vi "RG TAS v4c_Jamie_PIA.vi"() -> ()   [LabVIEW 2015]
uses:
  <vilib>/Analysis/2dsp.llb/Decimate (single shot, DBL).vi
  <vilib>/DAQmx/read.llb/DAQmx Read (Analog Wfm 1Chan NSamp).vi
  <vilib>/Analysis/baseanly.llb/Mean (DBL).vi
  Chaz TAS - DR/Sub VIs/Mono/global_Test.vi
  <vilib>/Instr/_visa.llb/VISA Configure Serial Port (Instr).vi
  Sub VIs/global tas.vi
  <vilib>/DAQmx/miscellaneous.llb/DAQmx Fill In Error Info.vi
  <vilib>/Utility/file.llb/Write To Spreadsheet File (DBL).vi
  <vilib>/Waveform/WDTOps.llb/WDT Index Channel DBL.vi
  <vilib>/Utility/file.llb/Write Delimited Spreadsheet (DBL).vi
  Program Files/National Instruments/LabVIEW 2014/instr.lib/Tektronix DPO MSO 2000 4000 Series/Tektronix DPO MSO 2000 4000 Series.lvlib
  <vilib>/Analysis/NI_AALPro.lvlib
  <vilib>/Analysis/NI_AALBase.lvlib
panel:
  in  "Inspect Traces":bool
  out "DAQ Loop":i32
  out "Scope Error Counter":i32
  out "Scope time axis":dbl[](array[numeric])
  in  "Stop acquisition":bool
  out "Grating":i32
  in  "2b - Spectrum":bool
  in  "2a - Kinetic":bool
  in  "Stop":bool
  out "Btrace Readout Counter":i32=2
  in  "Stop Btrace Measurement":bool
  out "Readout Counter":i32=2
  in  "Stop Measurement":bool
  in  "Calculate Output Method":T1(ring)=enum."Reflectance"
  in  "Parameters":T2(tab)
  in  "Shutter flow control":u16(ring) items=["None"=0, "XON/XOFF"=1, "RTS/CTS"=2, "DTR/DSR"=4]
  in  "Shutter stop bits":u16(ring)=10 items=["1.0"=10, "1.5"=15, "2.0"=20]
  in  "Shutter parity":u16(ring) items=["None", "Odd", "Even", "Mark", "Space"]
  in  "Shutter data bits":u16=8 min=5 max=8 step=1
  in  "Shutter VISA resource name":refnum<visa-resource-name>="COM1"
  in  "Shutter baud rate":u32=9600
  in  "Shutter open string":string="+100 10\n"
  in  "1 - Move Shutter":bool
  in  "3 - Move mono":bool
  out "Current wavelength (Oriel)":dbl format="%#_13g"
  in  "Monochromator Type":bool=TRUE
  out "Start Wavelength":dbl min=0.0 format="%.3f"
  out "End Wavelength":dbl=100.0 min=0.0 format="%.3f"
  out "Interval Wavelength":dbl=10.0 min=0.0 format="%.3f"
  out "Current Wavelength (PTI)":dbl=300.0 min=300.0 max=2000.0 step=1.0
  in  "Is IR":bool caption="Grating"
  in  "Mono VISA name":refnum<visa-resource-name>
  in  "Mono 2 VISA name":refnum<visa-resource-name>
  out "DAQ dt":dbl=5e-06
  in  "DAQ End Time (s)":dbl=1.0
  in  "DAQ rate":i32=1250000
  in  "DAQ Trigger Level (V)":dbl=0.2
  out "DAQ Number of Samples":dbl=10000.0
  in  "DAQ average number of points":dbl=50.0
  out "DAQ final number of points":dbl
  in  "DAQ Input Channel":tag="Dev1/ai0"
  in  "100% Reflectance Standard (V)":dbl=1.0
  in  "DAQ Card":enum16{"USB-6211", "USB-6251"}(ring)=enum."USB-6251"
  in  "DAQ Input Config":i32(ring)=10106 items=["default"=-1, "RSE"=10083, "NRSE"=10078, "Differential"=10106, "Pseudodifferential"=12529]
  in  "Record Length":u32(ring)=10 items=["1000 points"=1, "10k points"=10, "100k points"=100, "1M points"=1000, "5M points"=5000, "10M points"=10000]
  in  "Acquisition Type":u16(ring)=2 items=["Sample", "Peak Detect", "Hi Res", "Envelope", "Average"]
  in  "Scope average\nnumber of points":dbl=1.0
  in  "Averages on scope":i32=1
  in  "Using TDS Scope?":bool
  in  "CH2 Impedance":u16(ring) items=["1M", "75", "50"]
  in  "CH1 Impedance":u16(ring)=2 items=["1M", "75", "50"]
  in  "Scope VISA resource name":refnum<visa-resource-name>="USB0::0x0699::0x0410::C022077::INSTR"
  in  "Scope Timeout (ms)":u32=30000
  in  "Channel TAS (0: Channel 1)":u16(ring) caption="Channel TAS" items=["Channel 1", "Channel 2", "Channel 3", "Channel 4", "Math", "Reference A", "Reference B", "Reference C", "Reference D"]
  in  "Channel TPC (0: Channel 1)":u16(ring)=1 caption="Channel TPC" items=["Channel 1", "Channel 2", "Channel 3", "Channel 4", "Math", "Reference A", "Reference B", "Reference C", "Reference D"]
  in  "Scope Timebase (per div)":dbl=0.0001 format="%^#_3e"
  in  "Trigger Source":u16(ring)=1 items=["Channel 1", "Channel 2", "Channel 3", "Channel 4", "AC Line", "Aux", "Digital Channel 0", "Digital Channel 1", "Digital Channel 2", "Digital Channel 3", "Digital Channel 4", "Digital Channel 5", "Digital Channel 6", "Digital Channel 7", "Digital Channel 8", "Digital Channel 9", "Digital Channel 10", "Digital Channel 11", "Digital Channel 12", "Digital Channel 13", "Digital Channel 14", "Digital Channel 15", "RF"]
  out "Final number of\nscope points":dbl=10000.0
  in  "Vertical Coupling TAS (1: DC)":u16(ring)=1 caption="Vertical Coupling TAS" items=["AC", "DC", "Ground"]
  in  "Probe Attenuation TAS (10.0)":dbl=1.0 caption="Probe Attenuation TAS"
  in  "Bandwidth CHTAS (0: FULL)":i32(ring) caption="Bandwidth CH TAS" items=["FULL", "250 MHz", "150 MHz", "20 MHz"]
  in  "Vertical Offset CH TAS (0.0 divs)":dbl caption="Vertical Offset CH TAS (in V)"
  in  "Vertical Range CH TAS (10.0 V)":dbl=0.5 caption="Vertical Range CH TAS"
  in  "Trigger Level (V)":dbl=0.25
  in  "Vertical Coupling TPC (1: DC)":u16(ring)=1 caption="Vertical Coupling TPC" items=["AC", "DC", "Ground"]
  in  "Probe Attenuation TPC (1.0)":dbl=1.0 caption="Probe Attenuation TPC"
  in  "Vertical Range TPC (10.0 V)":dbl=0.2 caption="Vertical Range TPC"
  in  "Bandwidth CH TPC (0: FULL)":i32(ring) caption="Bandwidth CH TPC" items=["FULL", "250 MHz", "150 MHz", "20 MHz"]
  in  "Vertical Offset CH TPC (0.0 divs)":dbl caption="Vertical Offset CH TPC (in V)"
  in  "TPC Multiplication factor":dbl=1.0
  out "Number of scope readouts":i32
  in  "Scope Channel Read":bool
  in  "LED on (s)":dbl
  in  "LED off (s)":dbl
  in  "PIA Mode":bool
  in  "LEDs (constant irrad.)":bool caption="LEDs"
  in  "DAQ LED line":string="Dev1/port1/line0"
  in  "Control LEDs?":bool
  out "Scope pretrigger points":dbl=1000.0
  out "Scope CH1 DOD data (A-B final)":waveform(dbl)(graph)
  out "Scope CH1 DOD data (A final)":waveform(dbl)(graph)={"t0"=timestamp(-4.0000000000040004e-05 s since 1904-01-01), "dt"=4.0000000000000003e-07, "Y"=array[10000 elements]}
  out "Scope CH2 data (final)":waveform(dbl)(graph)={"t0"=timestamp(-4.0000000000040004e-05 s since 1904-01-01), "dt"=4.0000000000000003e-07, "Y"=array[10000 elements]}
  out "DAQ DOD data (final)":waveform(dbl)(graph)={"t0"=timestamp(0 s since 1904-01-01), "dt"=5e-06, "Y"=array[10000 elements]}
  out "B trace (Channel1)":waveform(dbl)(graph)
  in  "Amplification Factor":dbl=400.0
  out "Background level (on Amp)":dbl=30.577247161746392
  out "Background level (V)":dbl=0.08993307988748939
  in  "Trace B ?":bool=TRUE
  out "Folder Created":bool
  in  "Sample Name":string="Sample"
  in  "TAS2014  Path":path=path "D:/Solar Fuels Data" caption="Folder"
  out "Path to Files":path=path "D:/Solar Fuels Data/Sample"
  out "Scope Average Channel2":waveform(dbl)(graph)={"t0"=timestamp(-4.0000000000040004e-05 s since 1904-01-01), "dt"=4.0000000000000003e-07, "Y"=array[10000 elements]}
  out "Scope Average Channel1":waveform(dbl)(graph)={"t0"=timestamp(-4.0000000000040004e-05 s since 1904-01-01), "dt"=4.0000000000000003e-07, "Y"=array[10000 elements]}
  out "DAQ Average Data":waveform(dbl)(graph)={"t0"=timestamp(0 s since 1904-01-01), "dt"=5e-06, "Y"=array[10000 elements]}
  in  "Number of Averages":i32=32
  out "DAQ Live Data":waveform(dbl)(graph)={"t0"=timestamp(0 s since 1904-01-01), "dt"=4.999999999999959e-06, "Y"=array[10000 elements]}
  # "Acquisition"
  # "Format: +100\\s20\\n OR \\F3\\002\\C1"
  # "Set COM ports for PTI\nmonochromators. If there\nis only 1 monochromator\npresent, leave Mono 2\nVISA name empty."
  # "DAQ Controls"
  # "DAQ Indicators"
  # "(Max = 250k/1.25M for\n6211/6251 DAQ cards)"
  # "Default is differential (connected ports are 15 and 16 on DAQ card).\n* For CH-TAS, input config should be RSE."
  # "Recommended Parameters for Different Scope Models"
  # "DPO3012"
  # "Record Length = 10k\nScope average number of points = 1"
  # "Acquisition Type = Hi Res\nAverages on scope = 1"
  # "DPO2012B"
  # "Record Length = 1M\nScope average number of points = 100"
  # "Acquisition Type = Average\nAverages on scope = 4"
  # "TDS3012C"
  # "Record Length = 10k\nScope average number of points = 1"
  # "Acquisition Type = Sample\nAverages on scope = 1"
  # "Channel 1"
  # "Channel 2"
  # "* For DPO2012B, impedance must be 1M for both channels!"
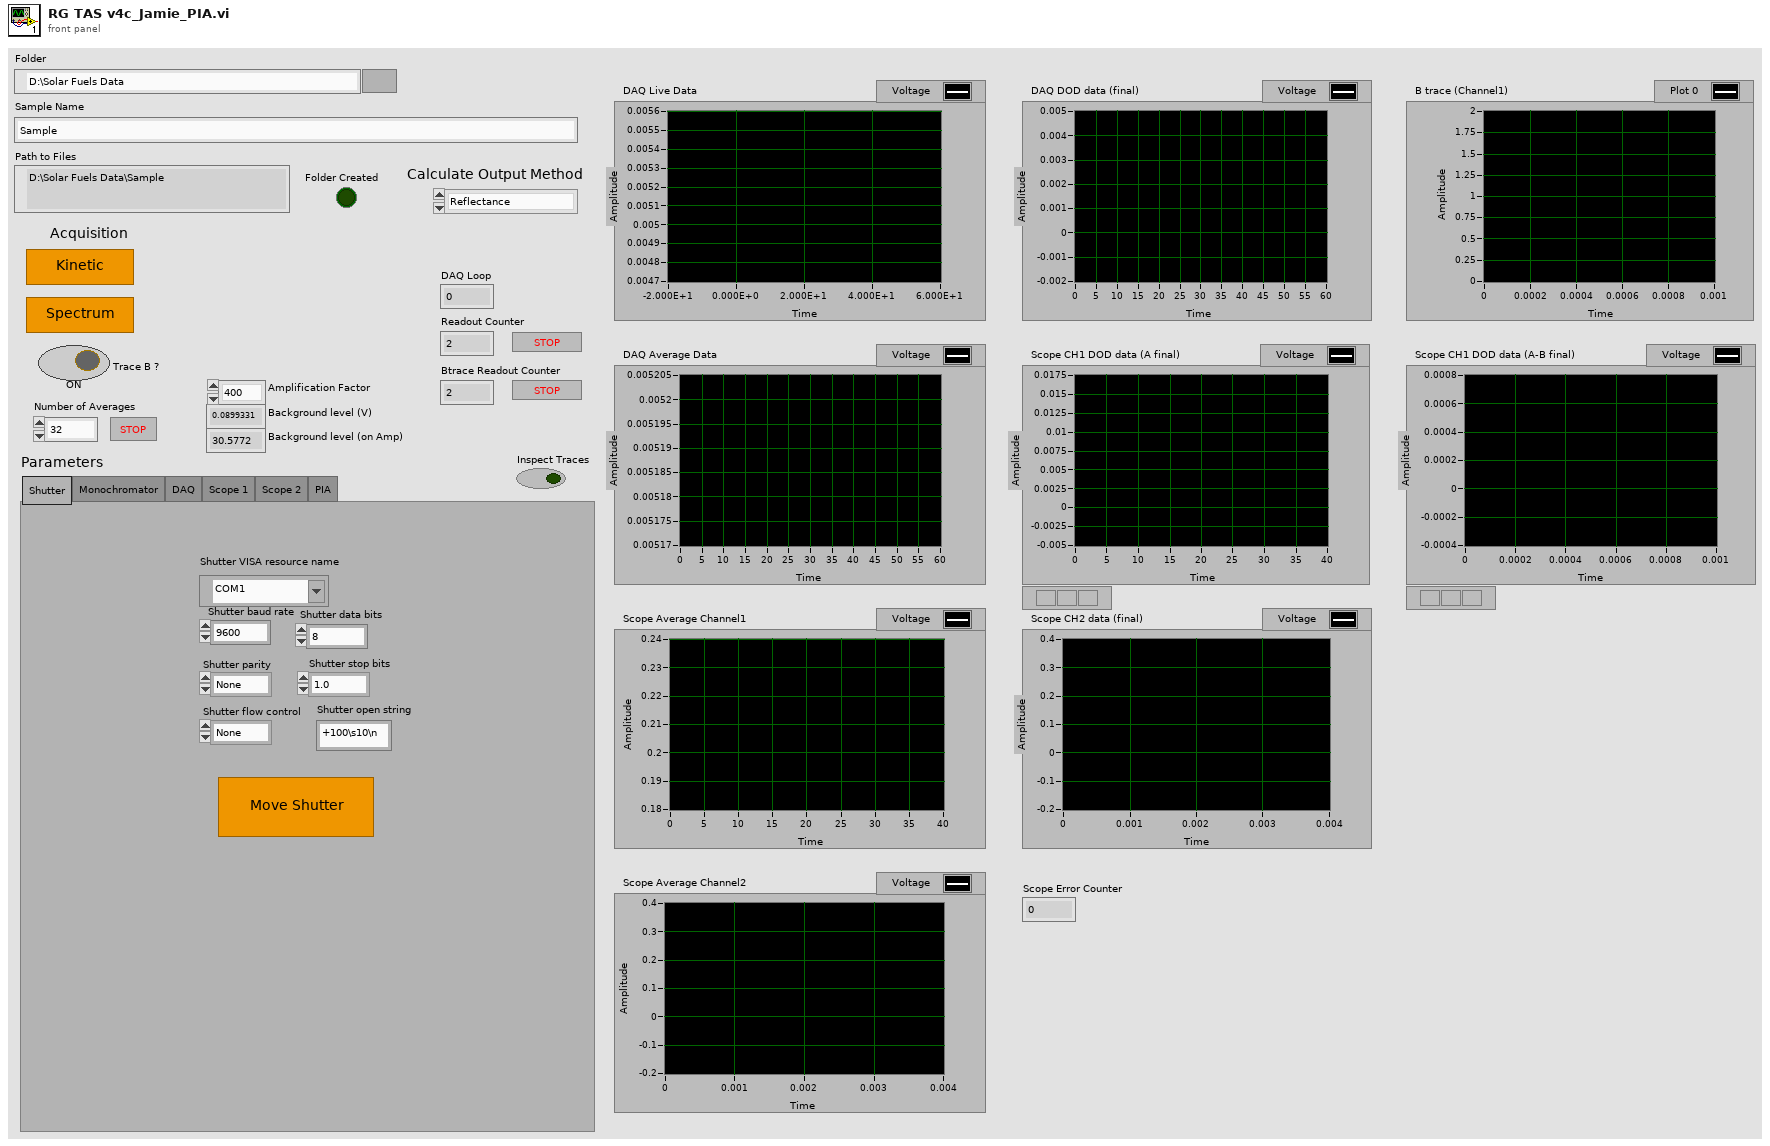
[diagram p1: front panel]
types:
  T1 = enum16{"Transmission", "Reflectance", "Kubelka-Munk"}
  T2 = enum32{"Shutter", "Monochromator", "DAQ", "Scope 1", "Scope 2", "PIA"}
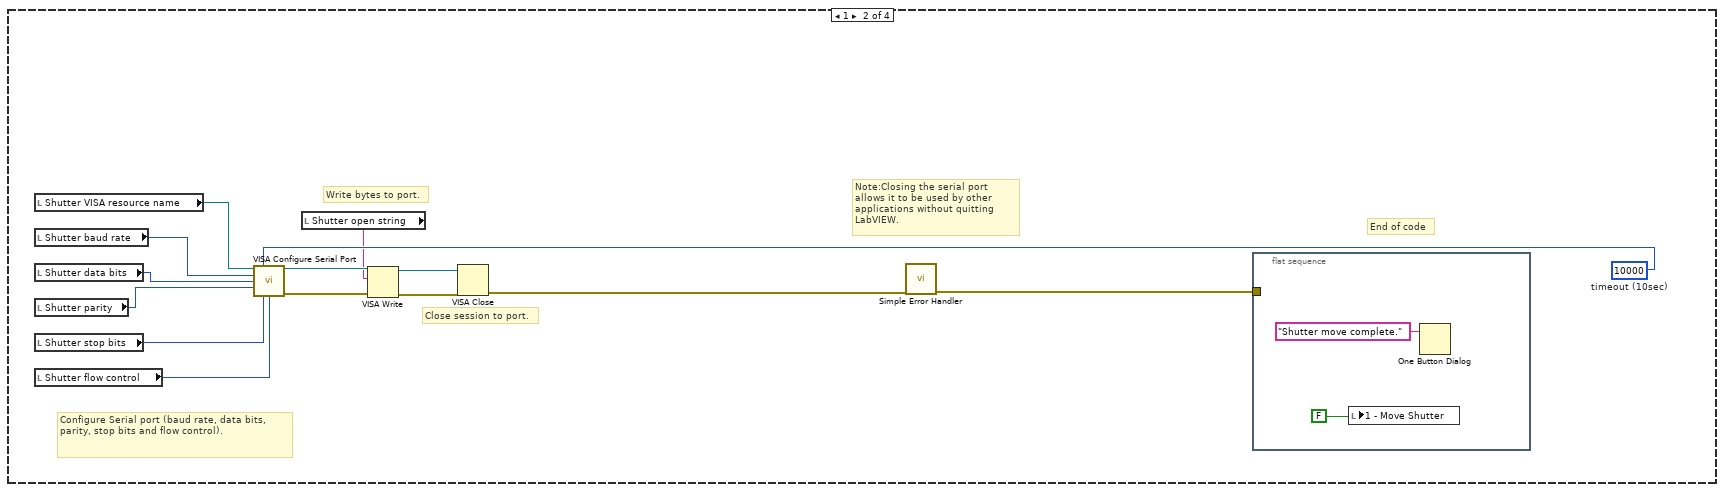
[diagram p4: hidden frame]
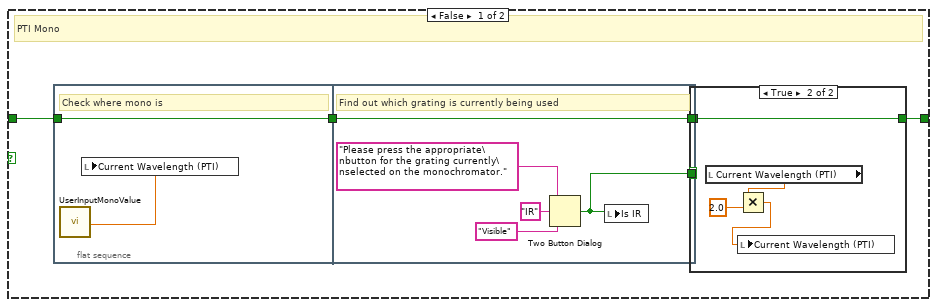
[diagram p5: hidden frame]
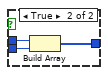
[diagram p8: hidden frame]
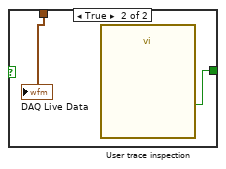
[diagram p9: hidden frame]
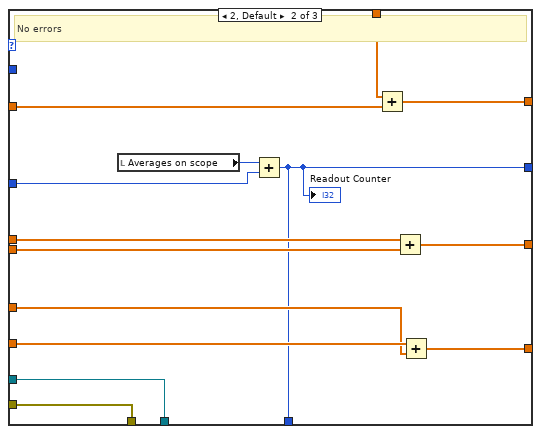
[diagram p11: hidden frame]
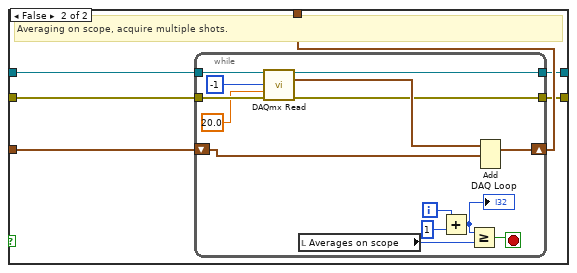
[diagram p13: hidden frame]
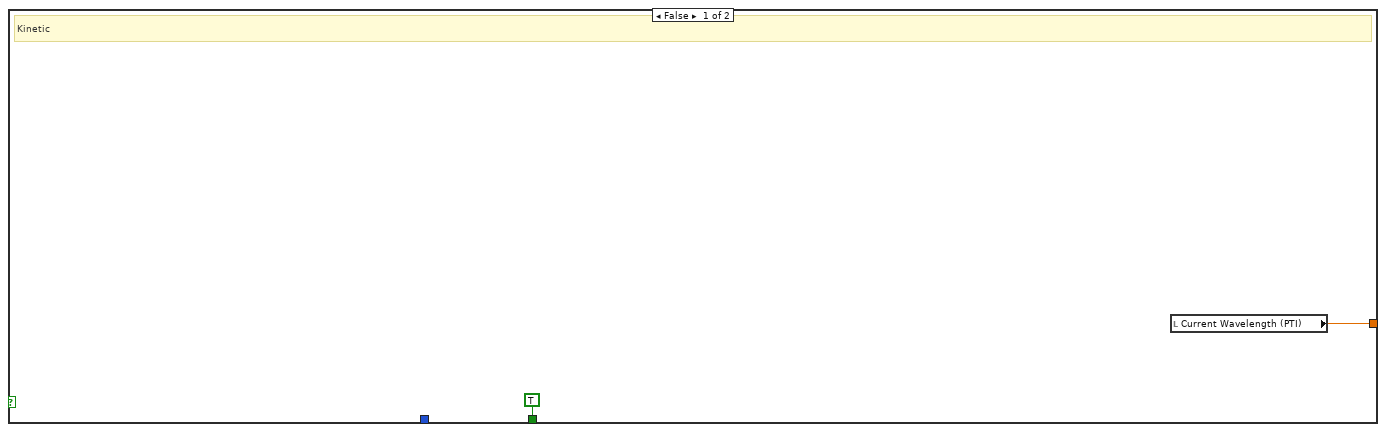
[diagram p14: hidden frame]
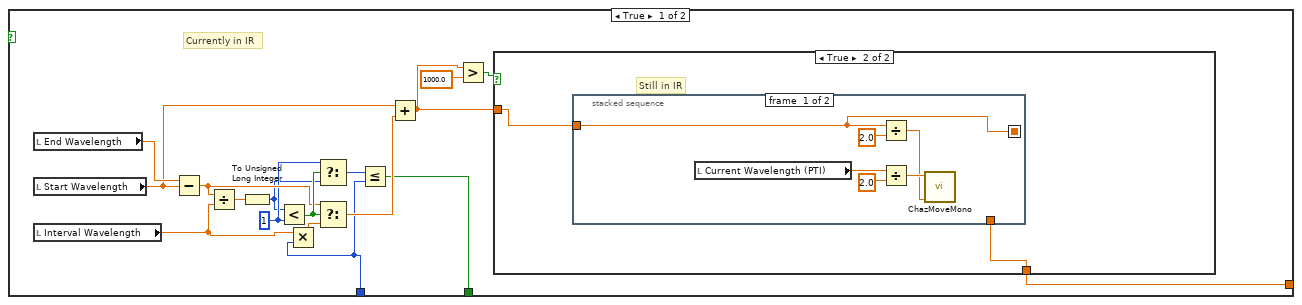
[diagram p15: hidden frame]
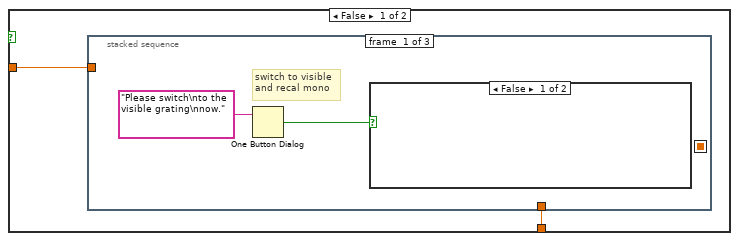
[diagram p16: hidden frame]
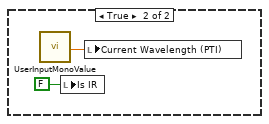
[diagram p17: hidden frame]
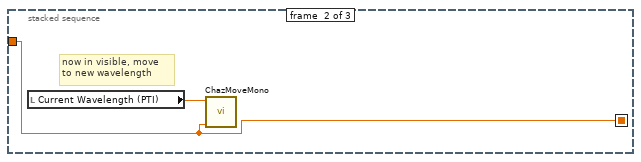
[diagram p18: hidden frame]
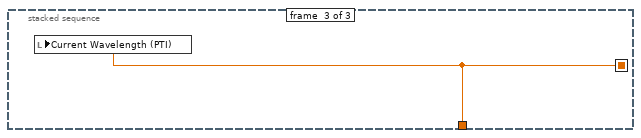
[diagram p19: hidden frame]
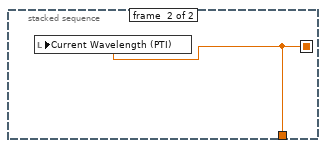
[diagram p20: hidden frame]
diagram:
  n1 = while {
    stop <- "Stop" stop-if-true
    # "True = Oriel"
    n2 = Or(x="2a - Kinetic", y="2b - Spectrum") -> (x .or. y?=w6:bool)
    n3 = Build Array(FALSE, "1 - Move Shutter", w6, "3 - Move mono") -> (w11:bool[])
    n4 = Search 1D Array(1D array=w11, element=TRUE) -> (index of element=w4:i32)  [unwired: 1 in]
    n5 = flat-sequence {
      tunnel: w4 -> [w37]
      tunnel: [w37] -> w3
      tunnel: "Monochromator Type" -> [w15]
      tunnel: [w15] -> w1
      frame #0 {
        # "Calculate DAQ parameters"
        # "Calculate Scope Parameters"
        n6 = case shown="True" "Control LEDs?" {
          frame False {
          }
          frame True {
            n7 = call "RG DAQ control for PIA.vi"("lines"="DAQ LED line", "Initial value"="LEDs (constant irrad.)") -> ()  [unwired: 10 in]
          }
        }
        n8 = Multiply(x="DAQ End Time (s)", y=1.1) -> (x*y=w16:dbl)
        n9 = Multiply(x="Record Length", y=u32 1000) -> (x*y=w25:u32)
        n10 = Multiply(x="DAQ rate", y=w16) -> (x*y=w24:dbl)
        "DAQ Number of Samples" <- w24
        n11 = Reciprocal(x="DAQ rate") -> (1/x=→"DAQ dt":dbl)
        n12 = Divide(x="Number of Averages", y="Averages on scope") -> (x/y=→"Number of scope readouts":dbl)
        n13 = Divide(x=w25, y="Scope average\nnumber of points") -> (x/y=w29:dbl)
        "Final number of\nscope points" <- w29
        n14 = Divide(x=w29, y=10.0) -> (x/y=→"Scope pretrigger points":dbl)
        n15 = Wait (ms)(milliseconds to wait=u32 1000) -> ()  [unwired: 1 out]
        n16 = Divide(x=w24, y="DAQ average number of points") -> (x/y=→"DAQ final number of points":dbl)
        n17 = global write "global_Test.vi" "Mono VISA name"("Mono VISA name") -> ()
        n18 = global write "global_Test.vi" "Mono 2 VISA name"("Mono 2 VISA name") -> ()
      }
    }
    n19 = case shown="2" w3 {
      tunnel: w1 -> [_ _ w56 w1010]
      frame 0, Default {
      }
      frame 1 {
        w48 = u32 10000  # timeout (10sec)
        # "End of code"
        # "Note:Closing the serial port allows it to be used by other applications without quitting LabVIEW."
        # "Close session to port."
        # "Configure Serial port (baud rate, data bits, parity, stop bits and flow control)."
        # "Write bytes to port."
        n20 = local read "Shutter VISA resource name"() -> (w47:refnum<visa-resource-name>)
        n21 = local read "Shutter baud rate"() -> (w46:u32)
        n22 = local read "Shutter data bits"() -> (w45:u16)
        n23 = local read "Shutter parity"() -> (w44:u16)
        n24 = local read "Shutter stop bits"() -> (w43:u16)
        n25 = local read "Shutter flow control"() -> (w42:u16)
        n26 = call-poly "VISA Configure Serial Port"("VISA resource name"=w47, "timeout (10sec)"=w48, "baud rate (9600)"=w46, "data bits (8)"=w45, "parity (0:none)"=w44, "stop bits (10: 1 bit)"=w43, "flow control (0:none)"=w42) -> ("VISA resource name out"=w49:refnum<visa-resource-name>, "error out"=w50:errorcluster)  [unwired: 2 in, 5 out]
        n27 = local read "Shutter open string"() -> (w41:string)
        n28 = VISA Write(VISA resource name=w49, write buffer=w41, error in (no error)=w50) -> (VISA resource name out=w52:refnum<visa-resource-name>, error out=w53:errorcluster)  [unwired: 1 out]
        n29 = VISA Close(VISA resource name=w52, error in (no error)=w53) -> (error out=w51:errorcluster)
        n30 = call <vilib>:"Simple Error Handler.vi"("error in (no error)"=w51) -> ("error out"=w40:errorcluster)  [unwired: 1 in, 7 out]
        n31 = flat-sequence {
          tunnel: w40 -> [_]
          frame #0 {
            n32 = local write "1 - Move Shutter"(FALSE ("Move Shutter")) -> ()
            n33 = One Button Dialog(message="Shutter move complete.") -> ()  [unwired: 1 in, 1 out]
          }
        }
      }
      frame 2 {
        n34 = Build Path(base path="TAS2014  Path", name or relative path="Sample Name") -> (appended path=w67:path)
        n35 = call <vilib>:"Check if File or Folder Exists.vi"("path"=w67) -> ("file or folder exists?"=w66:bool, "dup path"=w65:path)  [unwired: 8 in, 1 out]
        n36 = case shown="True" w66 {
          tunnel: w65 -> [w1002 w1008]
          tunnel: [w1001 w1008] -> w60
          frame False {
            n37 = Create Folder(path (use dialog)=w1002) -> (created path=w1001:path)  [unwired: 2 in, 2 out]
            n38 = local write "Folder Created"(TRUE ("Folder Created")) -> ()
          }
          frame True {
            n39 = Two Button Dialog(message="Caution - folder already exists. Continue to overwrite data?", 1:"Yes, go for it!" ("F button name (\"Cancel\")"), 2:"No, help me!" ("T button name (\"OK\")")) -> (T button?=w1003:bool)
            n40 = local write "Folder Created"(FALSE ("Folder Created")) -> ()
            n41 = Stop(stop? (T)=w1003) -> ()
          }
        }
        "Path to Files" <- w60
        n42 = case shown="True" w56 {
          tunnel: w56 -> [w71 w86]
          tunnel: [w69 w85] -> w57
          frame False {
            # "PTI Mono"
            n43 = flat-sequence {
              tunnel: [w78] -> w72
              tunnel: w71 -> [w78]
              tunnel: w72 -> [w84]
              tunnel: [w84] -> w70
              tunnel: [w80] -> w68
              frame #0 {
                # "Check where mono is"
                n44 = call "UserInputMonoValue.vi"() -> ("Monochromator readout"=w79:dbl)  [unwired: 17 in, 2 out]
                n45 = local write "Current Wavelength (PTI)"(w79) -> ()
              }
              frame #1 {
                # "Find out which grating is currently being used"
                n46 = Two Button Dialog(message="Please press the appropriate\nbutton for the grating currently\nselected on the monochromator.", 1:"Visible" ("F button name (\"Cancel\")"), 2:"IR" ("T button name (\"OK\")")) -> (T button?=w80:bool)
                n47 = local write "Is IR"(w80) -> ()
              }
            }
            n48 = case shown="True" w68 {
              tunnel: w70 -> [w73 w77]
              tunnel: [w73 w77] -> w69
              frame False {
              }
              frame True {
                n49 = local read "Current Wavelength (PTI)"() -> (w75:dbl)
                n50 = Multiply(x=w75, y=2.0) -> (x*y=w74:dbl)
                n51 = local write "Current Wavelength (PTI)"(w74) -> ()
              }
            }
          }
          frame True {
            # "Oriel Mono"
            n52 = flat-sequence {
              tunnel: w86 -> [w90]
              tunnel: [w90] -> w85
              frame #0 {
                n53 = call "m_open.vi"() -> ("error out"=w91:errorcluster, "configuration file path copy"=w87:path)  [unwired: 2 in]
                n54 = call "GetWave.vi"("error in (no error)"=w91) -> ("error out"=w89:errorcluster, "Present Wavelength"=w88:dbl)  [unwired: 1 in]
                n55 = call "m_close.vi"("error in (no error)"=w89, "configuration file path"=w87) -> ()  [unwired: 2 out]
                n56 = local write "Current wavelength (Oriel)"(w88) -> ()
              }
            }
          }
        }
        n57 = local read "2b - Spectrum"() -> (w62:bool)
        n58 = global write "global tas.vi" "Root Path"(w60) -> ()
        n59 = case shown="True" w62 {
          tunnel: w60 -> [w95 w96]
          tunnel: [w95 w96] -> w58
          frame False {
          }
          frame True {
            n60 = call "RG Get Spectrum Wavelengths.vi"() -> ("Wavelength interval"=→"Interval Wavelength":i32, "End wavelength"=→"End Wavelength":i32, "Start wavelength"=→"Start Wavelength":i32)  [unwired: 9 in]
          }
        }
        n61 = flat-sequence {
          tunnel: [w92] -> w59
          tunnel: w58 -> [_]
          frame #0 {
            n62 = call "Prompt User for Input"() -> ("yes"=w92:bool)  [unwired: 18 in, 1 out]
          }
        }
        n63 = while {
          tunnel: [w207] -> w61
          tunnel: w59 -> [w202]
          tunnel: w57 -> [w195]
          i -> [w196]
          stop <- w225 stop-if-true
          w284 = TRUE  # Reset (True)
          w163 = 0
          w287 = FALSE  # ID Query (True)
          w320 = FALSE  # Enable Continuous Acquisition Mode (True)
          # "Some Maths to automatically output a stitched Scope-DAQ trace"
          # "Scope t0"
          # "Scope dt"
          # "DAQ index to make\nsure DAQ acquisition\nis finished before\ndoing B trace."
          # "Scope time\naxis"
          # "Scope time axis"
          # "Current wavelength"
          # "Current Wavelength"
          # "Make sure the 20s is waited before starting to acquire the data if shutter moves."
          # "Set time so that trigger\nis at t = 0"
          # "Get pre laser light level"
          # "Change cases for old TDS scope models because of differences in programming commands."
          # "Get pre laser light level (V) for DAQ and Scope"
          # "Disable time delay"
          # "Configure Timebase"
          # "Disable continous acquisition"
          # "Configure Trigger"
          # "If reading 2 channels, combine Channel A\n and Channel B so that both channels are read"
          # "Configure Channel B"
          # "Configure Channel A"
          # "Check the initial position of the shutter, and move if Doing Trace B and Spectrum"
          n64 = local read "2b - Spectrum"() -> (w199:bool)
          n65 = case shown="False" w195 {
            tunnel: [w561 w652] -> w224
            tunnel: [w558 w651] -> w222
            tunnel: [w560 w650] -> w206
            tunnel: w199 -> [w562 w649]
            tunnel: w196 -> [w563 w648]
            frame False {
              # "PTI Monochromator"
              n66 = flat-sequence {
                tunnel: w563 -> [w567]
                tunnel: w562 -> [w566]
                tunnel: [w565] -> w561
                tunnel: [w564] -> w559
                tunnel: [w647] -> w560
                tunnel: w559 -> [w647]
                tunnel: [w646] -> w558
                frame #0 {
                  n67 = case shown="True" w566 {
                    tunnel: w567 -> [_ w572]
                    tunnel: [TRUE w571] -> w565
                    tunnel: [w569 w570] -> w564
                    frame False {
                      # "Kinetic"
                      n68 = local read "Current Wavelength (PTI)"() -> (w569:dbl)
                    }
                    frame True {
                      # "Spectrum"
                      n69 = case shown="False" "Is IR" {
                        tunnel: w572 -> [w576 w612]
                        tunnel: [w577 w611] -> w571
                        tunnel: [w575 w610] -> w570
                        frame True {
                          w585 = u32 1 ("y")
                          # "Currently in IR"
                          n70 = local read "End Wavelength"() -> (w583:dbl)
                          n71 = local read "Start Wavelength"() -> (w581:dbl)
                          n72 = local read "Interval Wavelength"() -> (w578:dbl)
                          n73 = Subtract(x=w583, y=w581) -> (x-y=w586:dbl)
                          n74 = Divide(x=w586, y=w578) -> (x/y=w588:dbl)
                          n75 = To Unsigned Long Integer(number=w588) -> (unsigned 32bit integer=w584:u32)
                          n76 = Less?(x=w584, y=w585) -> (x < y?=w587:bool)
                          n77 = Multiply(x=w578, y=w576) -> (x*y=w579:dbl)
                          n78 = Select(t=w585, s=w587, f=w584) -> (s? t:f=w582:u32)
                          n79 = Select(t=w586, s=w587, f=w579) -> (s? t:f=w580:dbl)
                          n80 = Less Or Equal?(x=w582, y=w576) -> (x <= y?=w577:bool)
                          n81 = Add(x=w581, y=w580) -> (x+y=w574:dbl)
                          n82 = Greater?(x=w574, y=1000.0) -> (0:w589:bool)
                          n83 = case shown="True" w589 {
                            tunnel: [w592 w601] -> w575
                            tunnel: w574 -> [w591 w600]
                            frame False {
                              n84 = stacked-sequence {
                                seq-local: [_ w597 _] -> [_ _ w599]
                                tunnel: [_ _ w599] -> w592
                                tunnel: w591 -> [_ w597 _]
                                frame #0 {
                                # "switch to visible\nand recal mono"
                                n85 = One Button Dialog(message="Please switch\nto the visible grating\nnow.") -> (true=w593:bool)  [unwired: 1 in]
                                n86 = case shown="False" w593 {
                                frame False {
                                }
                                frame True {
                                n87 = call "UserInputMonoValue.vi"() -> ("Monochromator readout"=w595:dbl)  [unwired: 17 in, 2 out]
                                n88 = local write "Is IR"(FALSE ("Is IR")) -> ()
                                n89 = local write "Current Wavelength (PTI)"(w595) -> ()
                                }
                                }
                                }
                                frame #1 {
                                # "now in visible, move \nto new wavelength"
                                n90 = local read "Current Wavelength (PTI)"() -> (w598:dbl)
                                n91 = call "ChazMoveMono.vi"("Move to"=w597, "Current"=w598) -> ()  [unwired: 8 in, 2 out]
                                }
                                frame #2 {
                                n92 = local write "Current Wavelength (PTI)"(w599) -> ()
                                }
                              }
                            }
                            frame True {
                              # "Still in IR"
                              n93 = stacked-sequence {
                                seq-local: [w602 _] -> [_ w608]
                                tunnel: [_ w608] -> w601
                                tunnel: w600 -> [w602 _]
                                frame #0 {
                                n94 = local read "Current Wavelength (PTI)"() -> (w607:dbl)
                                n95 = Divide(x=w602, y=2.0) -> (x/y=w603:dbl)
                                n96 = Divide(x=w607, y=2.0) -> (x/y=w604:dbl)
                                n97 = call "ChazMoveMono.vi"("Move to"=w603, "Current"=w604) -> ()  [unwired: 8 in, 2 out]
                                }
                                frame #1 {
                                n98 = local write "Current Wavelength (PTI)"(w608) -> ()
                                }
                              }
                            }
                          }
                        }
                        frame False {
                          w620 = u32 1 ("y")
                          # "Currently in Visible"
                          n99 = local read "End Wavelength"() -> (w618:dbl)
                          n100 = local read "Start Wavelength"() -> (w616:dbl)
                          n101 = local read "Interval Wavelength"() -> (w613:dbl)
                          n102 = Subtract(x=w618, y=w616) -> (x-y=w621:dbl)
                          n103 = Divide(x=w621, y=w613) -> (x/y=w623:dbl)
                          n104 = To Unsigned Long Integer(number=w623) -> (unsigned 32bit integer=w619:u32)
                          n105 = Less?(x=w619, y=w620) -> (x < y?=w622:bool)
                          n106 = Multiply(x=w613, y=w612) -> (x*y=w614:dbl)
                          n107 = Select(t=w620, s=w622, f=w619) -> (s? t:f=w617:u32)
                          n108 = Select(t=w621, s=w622, f=w614) -> (s? t:f=w615:dbl)
                          n109 = Less Or Equal?(x=w617, y=w612) -> (x <= y?=w611:bool)
                          n110 = Add(x=w616, y=w615) -> (x+y=w609:dbl)
                          n111 = Greater?(x=w609, y=1000.0) -> (0:w624:bool)
                          n112 = case shown="False" w624 {
                            tunnel: [w627 w632] -> w610
                            tunnel: w609 -> [w626 w631]
                            frame False {
                              # "Still in Visible"
                              n113 = stacked-sequence {
                                seq-local: [w628 _] -> [_ w630]
                                tunnel: [_ w630] -> w627
                                tunnel: w626 -> [w628 _]
                                frame #0 {
                                n114 = local read "Current Wavelength (PTI)"() -> (w629:dbl)
                                n115 = call "ChazMoveMono.vi"("Move to"=w628, "Current"=w629) -> ()  [unwired: 8 in, 2 out]
                                }
                                frame #1 {
                                n116 = local write "Current Wavelength (PTI)"(w630) -> ()
                                }
                              }
                            }
                            frame True {
                              n117 = stacked-sequence {
                                seq-local: [_ w639 _] -> [_ _ w645]
                                tunnel: [_ _ w645] -> w632
                                tunnel: w631 -> [_ w639 _]
                                frame #0 {
                                # "switch to IR\nand recal mono"
                                n118 = One Button Dialog(message="Please switch\nto the IR grating\nnow.") -> (true=w633:bool)  [unwired: 1 in]
                                n119 = case shown="True" w633 {
                                frame False {
                                }
                                frame True {
                                n120 = call "UserInputMonoValue.vi"() -> ("Monochromator readout"=w637:dbl)  [unwired: 17 in, 2 out]
                                n121 = local write "Is IR"(TRUE ("Is IR")) -> ()
                                n122 = Multiply(x=w637, y=2.0) -> (x*y=w635:dbl)
                                n123 = local write "Current Wavelength (PTI)"(w635) -> ()
                                }
                                }
                                }
                                frame #1 {
                                # "now in IR, move \nto new wavelength"
                                n124 = local read "Current Wavelength (PTI)"() -> (w642:dbl)
                                n125 = Divide(x=w639, y=2.0) -> (x/y=w640:dbl)
                                n126 = Divide(x=w642, y=2.0) -> (x/y=w641:dbl)
                                n127 = call "ChazMoveMono.vi"("Move to"=w640, "Current"=w641) -> ()  [unwired: 8 in, 2 out]
                                }
                                frame #2 {
                                n128 = local write "Current Wavelength (PTI)"(w645) -> ()
                                }
                              }
                            }
                          }
                        }
                      }
                    }
                  }
                }
                frame #1 {
                  n129 = call <vilib>:"General Error Handler.vi"() -> ("error out"=w646:errorcluster)  [unwired: 11 in, 4 out]
                }
              }
            }
            frame True {
              # "Oriel Monochromator"
              n130 = case shown="False" w649 {
                tunnel: [TRUE w682] -> w652
                tunnel: w648 -> [_ w669]
                tunnel: [w654 w667] -> w651
                tunnel: [w653 w666] -> w650
                frame False {
                  # "B trace OFF"
                  n131 = call "m_open.vi"() -> ("error out"=w656:errorcluster, "configuration file path copy"=w655:path)  [unwired: 2 in]
                  n132 = call "GetWave.vi"("error in (no error)"=w656) -> ("error out"=w664:errorcluster, "Present Wavelength"=w653:dbl)  [unwired: 1 in]
                  "Current wavelength (Oriel)" <- w653
                  n133 = Less Or Equal?(x=w653, y=590.0) -> (x <= y?=w663:bool)
                  n134 = Select(t=1.0, s=w663, f=2.0) -> (s? t:f=w660:dbl)
                  n135 = call "setgrat.vi"("error in (no error)"=w664, "Grating"=w660) -> ("error out"=w661:errorcluster)  [unwired: 1 in]
                  n136 = call "gowave.vi"("error in (no error)"=w661, "Destination Wavelength"=w653) -> ("error out"=w662:errorcluster)
                  n137 = call "m_close.vi"("error in (no error)"=w662, "configuration file path"=w655) -> ("error out"=w654:errorcluster)  [unwired: 1 out]
                }
                frame True {
                  w686 = u32 1 ("y")
                  # "B trace ON"
                  n138 = local read "End Wavelength"() -> (w684:dbl)
                  n139 = local read "Start Wavelength"() -> (w673:dbl)
                  n140 = local read "Interval Wavelength"() -> (w670:dbl)
                  n141 = Subtract(x=w684, y=w673) -> (x-y=w687:dbl)
                  n142 = Divide(x=w687, y=w670) -> (x/y=w689:dbl)
                  n143 = To Unsigned Long Integer(number=w689) -> (unsigned 32bit integer=w685:u32)
                  n144 = Less?(x=w685, y=w686) -> (x < y?=w688:bool)
                  n145 = Multiply(x=w670, y=w669) -> (x*y=w671:dbl)
                  n146 = Select(t=w686, s=w688, f=w685) -> (s? t:f=w683:u32)
                  n147 = Select(t=w687, s=w688, f=w671) -> (s? t:f=w672:dbl)
                  n148 = Less Or Equal?(x=w683, y=w669) -> (x <= y?=w682:bool)
                  n149 = Add(x=w673, y=w672) -> (x+y=w666:dbl)
                  n150 = call "m_open.vi"() -> ("error out"=w668:errorcluster, "configuration file path copy"=w681:path)  [unwired: 2 in]
                  n151 = Less Or Equal?(x=w666, y=590.0) -> (x <= y?=w674:bool)
                  n152 = local write "Current wavelength (Oriel)"(w666) -> ()
                  n153 = Select(t=1.0, s=w674, f=2.0) -> (s? t:f=w677:dbl)
                  n154 = call "setgrat.vi"("error in (no error)"=w668, "Grating"=w677) -> ("error out"=w676:errorcluster)  [unwired: 1 in]
                  n155 = call "gowave.vi"("error in (no error)"=w676, "Destination Wavelength"=w666) -> ("error out"=w675:errorcluster)
                  n156 = call "m_close.vi"("error in (no error)"=w675, "configuration file path"=w681) -> ("error out"=w667:errorcluster)  [unwired: 1 out]
                }
              }
            }
          }
          n157 = local read "Scope VISA resource name"() -> (w330:refnum<visa-resource-name>)
          n158 = local read "Trace B ?"() -> (w200:bool)
          n159 = And(x=w200, y=w199) -> (x .and. y?=w198:bool)
          n160 = Not Equal To 0?(x=w196) -> (x != 0?=w197:bool)
          n161 = And(x=w198, y=w197) -> (x .and. y?=w201:bool)
          n162 = Or(x=w202, y=w201) -> (x .or. y?=w203:bool)
          n163 = call "Initialize.vi"("error in (no error)"=w222, "Reset (True)"=w284, "ID Query (True)"=w287, "VISA resource name"=w330) -> ("error out"=w322:errorcluster, "VISA resource name out"=w321:refnum<visa-resource-name>)  [unwired: 6 in]
          n164 = local read "Scope Timeout (ms)"() -> (w157:u32)
          n165 = case shown="True" w203 {
            tunnel: [u32 0 ("millisecond timer value") w985] -> w142
            frame False {
            }
            frame True {
              w995 = u32 10000  # timeout (10sec)
              # "Note:Closing the serial port allows it to be used by other applications without quitting LabVIEW."
              # "Close session to port."
              # "Configure Serial port (baud rate, data bits, parity, stop bits and flow control)."
              # "Write bytes to port."
              n166 = call-poly "VISA Configure Serial Port"("VISA resource name"="Shutter VISA resource name", "timeout (10sec)"=w995, "baud rate (9600)"="Shutter baud rate", "data bits (8)"="Shutter data bits", "parity (0:none)"="Shutter parity", "stop bits (10: 1 bit)"="Shutter stop bits", "flow control (0:none)"="Shutter flow control") -> ("VISA resource name out"=w991:refnum<visa-resource-name>, "error out"=w990:errorcluster)  [unwired: 2 in, 5 out]
              n167 = VISA Write(VISA resource name=w991, write buffer="Shutter open string", error in (no error)=w990) -> (VISA resource name out=w988:refnum<visa-resource-name>, error out=w987:errorcluster)  [unwired: 1 out]
              n168 = VISA Close(VISA resource name=w988, error in (no error)=w987) -> (error out=w989:errorcluster)
              n169 = call <vilib>:"Simple Error Handler.vi"("error in (no error)"=w989) -> ()  [unwired: 1 in, 8 out]
              n170 = Wait (ms)(milliseconds to wait=u32 20000) -> (millisecond timer value=w985:u32)
            }
          }
          n171 = call "Configure Continuous Acquisition.vi"("error in (no error)"=w322, "Enable Continuous Acquisition Mode (T: Enable)"=w320, "VISA resource name"=w321) -> ("error out"=w161:errorcluster, "VISA resource name out"=w162:refnum<visa-resource-name>)  [unwired: 7 in]
          n172 = local read "Vertical Range CH TAS (10.0 V)"() -> (w315:dbl)
          n173 = local read "Vertical Offset CH TAS (0.0 divs)"() -> (w332:dbl)
          n174 = property class="Instr"(reference=w162, error in=w161, "General Settings:Timeout Value"=w157) -> (reference out=w160:refnum<visa-resource-name>, error out=w159:errorcluster)
          n175 = local read "Vertical Coupling TAS (1: DC)"() -> (w313:u16)
          n176 = local read "Bandwidth CHTAS (0: FULL)"() -> (w311:i32)
          n177 = local read "Probe Attenuation TAS (10.0)"() -> (w331:dbl)
          n178 = local read "Channel TAS (0: Channel 1)"() -> (w312:u16)
          n179 = Or(x=w224, y="Stop acquisition") -> (x .or. y?=w225:bool)
          n180 = local read "Vertical Offset CH TPC (0.0 divs)"() -> (w329:dbl)
          n181 = local read "Vertical Coupling TPC (1: DC)"() -> (w309:u16)
          n182 = local read "Probe Attenuation TPC (1.0)"() -> (w328:dbl)
          n183 = local read "Channel TPC (0: Channel 1)"() -> (w310:u16)
          n184 = local read "Vertical Range TPC (10.0 V)"() -> (w314:dbl)
          n185 = local read "Bandwidth CH TPC (0: FULL)"() -> (w308:i32)
          n186 = local read "Scope Timebase (per div)"() -> (w140:dbl)
          n187 = local read "Record Length"() -> (w305:u32)
          n188 = case shown="False" "Using TDS Scope?" {
            tunnel: w332 -> [w955 w983]
            tunnel: w331 -> [w954 w982]
            tunnel: w329 -> [w953 w981]
            tunnel: w328 -> [w952 w980]
            tunnel: w159 -> [w951 w979]
            tunnel: w160 -> [w950 w978]
            tunnel: w315 -> [w947 w975]
            tunnel: w314 -> [w946 w974]
            tunnel: w313 -> [w943 w971]
            tunnel: w312 -> [w942 w970]
            tunnel: w311 -> [w941 w969]
            tunnel: w310 -> [w940 w968]
            tunnel: w309 -> [w939 w967]
            tunnel: w308 -> [w938 w966]
            tunnel: w305 -> [w937 w965]
            tunnel: [w935 w963] -> w304
            tunnel: [w933 w961] -> w303
            tunnel: "CH1 Impedance" -> [w931 w959]
            tunnel: "CH2 Impedance" -> [w930 w958]
            tunnel: w140 -> [w929 w957]
            tunnel: 10.0 ("Position (10 %)") -> [w928 w956]
            frame True {
              n189 = call "RG Configure Channel TDS3012C.vi"("VISA resource name"=w950, "Input Impedance (0: 1M ohm)"=w931, "Channel (0: Channel 1)"=w942, "Vertical Coupling (1: DC)"=w943, "Probe Attenuation (1)"=w954, "error in (no error)"=w951, "Vertical Range (10.0 V)"=w947, "Vertical Offset (0.0 V)"=w955, "Bandwidth (0: FULL)"=w941) -> ("VISA resource name out"=w949:refnum<visa-resource-name>, "error out"=w948:errorcluster)  [unwired: 5 in]
              n190 = call "RG Configure Channel TDS3012C.vi"("VISA resource name"=w949, "Input Impedance (0: 1M ohm)"=w930, "Channel (0: Channel 1)"=w940, "Vertical Coupling (1: DC)"=w939, "Probe Attenuation (1)"=w952, "error in (no error)"=w948, "Vertical Range (10.0 V)"=w946, "Vertical Offset (0.0 V)"=w953, "Bandwidth (0: FULL)"=w938) -> ("VISA resource name out"=w944:refnum<visa-resource-name>, "error out"=w945:errorcluster)  [unwired: 5 in]
              n191 = call "RG Configure Timebase TDS3012C.vi"("Record Length (10: 10k points)"=w937, "error in (no error)"=w945, "Position (10 %)"=w928, "Timebase (0.0005 s)"=w929, "VISA resource name"=w944) -> ("error out"=w934:errorcluster, "VISA resource name out"=w936:refnum<visa-resource-name>)  [unwired: 5 in]
              n192 = call "RG Configure Delay TDS3012C.vi"("error in (no error)"=w934, "Enable Delay (T: Enable)"=FALSE, "VISA resource name"=w936) -> ("error out"=w933:errorcluster, "VISA resource name out"=w935:refnum<visa-resource-name>)  [unwired: 7 in]
            }
            frame False {
              n193 = call "Configure Channel.vi"("VISA resource name"=w978, "Input Impedance (0: 1M ohm)"=w959, "Channel (0: Channel 1)"=w970, "Vertical Coupling (1: DC)"=w971, "Probe Attenuation (1)"=w982, "error in (no error)"=w979, "Vertical Range (10.0 V)"=w975, "Vertical Offset (0.0 V)"=w983, "Bandwidth (0: FULL)"=w969) -> ("VISA resource name out"=w977:refnum<visa-resource-name>, "error out"=w976:errorcluster)  [unwired: 5 in]
              n194 = call "Configure Channel.vi"("VISA resource name"=w977, "Input Impedance (0: 1M ohm)"=w958, "Channel (0: Channel 1)"=w968, "Vertical Coupling (1: DC)"=w967, "Probe Attenuation (1)"=w980, "error in (no error)"=w976, "Vertical Range (10.0 V)"=w974, "Vertical Offset (0.0 V)"=w981, "Bandwidth (0: FULL)"=w966) -> ("VISA resource name out"=w972:refnum<visa-resource-name>, "error out"=w973:errorcluster)  [unwired: 5 in]
              n195 = call "Configure Timebase.vi"("Record Length (10: 10k points)"=w965, "error in (no error)"=w973, "Position (10 %)"=w956, "Timebase (0.0005 s)"=w957, "VISA resource name"=w972) -> ("error out"=w962:errorcluster, "VISA resource name out"=w964:refnum<visa-resource-name>)  [unwired: 5 in]
              n196 = call "Configure Delay.vi"("error in (no error)"=w962, "Enable Delay (T: Enable)"=FALSE, "VISA resource name"=w964) -> ("error out"=w961:errorcluster, "VISA resource name out"=w963:refnum<visa-resource-name>)  [unwired: 7 in]
            }
          }
          n197 = Multiply(x=w140, y=1800.0) -> (x*y=w138:dbl)
          n198 = flat-sequence {
            tunnel: [w340] -> w156
            tunnel: [w339] -> w155
            tunnel: [w338] -> w149
            tunnel: w142 -> [w337]
            tunnel: [w337] -> w141
            frame #0 {
              # "DAQ Setup acquisition"
              n199 = local read "DAQ Number of Samples"() -> (w341:dbl)
              n200 = local read "DAQ Trigger Level (V)"() -> (w348:dbl)
              n201 = local read "DAQ Input Channel"() -> (w349:tag)
              n202 = local read "DAQ rate"() -> (w342:i32)
              n203 = call "RG Configure DAQ auto Max input scale.vi"("input terminal configuration"="DAQ Input Config", "DAQ Card Type"="DAQ Card", "Sampling rate"=w342, "DAQ Trigger Level"=w348, "physical channel"=w349, "number of samples"=w341) -> ("error out"=w340:errorcluster, "task out"=w339:refnum<k21>)  [unwired: 4 in]
              n204 = Reciprocal(x=w342) -> (1/x=w343:dbl)
              n205 = Initialize Array(0.0 ("element"), w341) -> (w344:dbl[])
              n206 = Bundle By Name("Y"=w344, "dt"=w343) -> (w338:waveform(dbl))  [unwired: 1 in]
            }
          }
          n207 = Max & Min(x=w138, y=700.0) -> (max(x,y)=w136:dbl)  [unwired: 1 out]
          n208 = local read "Trigger Level (V)"() -> (w307:dbl)
          n209 = local read "Trigger Source"() -> (w306:u16)
          n210 = local read "DAQ final number of points"() -> (w168:dbl)
          n211 = case shown="False" "Scope Channel Read" {
            tunnel: [w350 w354] -> w323
            tunnel: w312 -> [w351 w353]
            tunnel: w310 -> [_ w352]
            frame False {
              n212 = Build Array(w351) -> (w350:u16[])
            }
            frame True {
              n213 = Build Array(w353, w352) -> (w354:u16[])
            }
          }
          n214 = local read "Averages on scope"() -> (w230:i32)
          n215 = call "RG Configure Trigger (Edge).vi"("VISA resource name"=w304, "Trigger Source (0: Channel 1)"=w306, "Trigger Level (0.0 V)"=w307, "error in (no error)"=w303) -> ("VISA resource name out"=w299:refnum<visa-resource-name>, "error out"=w300:errorcluster)  [unwired: 10 in]
          n216 = local read "Final number of\nscope points"() -> (w293:dbl)
          n217 = call "Configure Acquisition.vi"("error in (no error)"=w300, "Number of Waveform Acquisitions (16)"=w230, "Acquisition Type (0: Sample)"="Acquisition Type", "VISA resource name"=w299) -> ("error out"=w133:errorcluster, "VISA resource name out"=w135:refnum<visa-resource-name>)  [unwired: 6 in]
          n218 = local write "Scope Error Counter"(w163) -> ()
          n219 = flat-sequence {
            tunnel: w135 -> [w336]
            tunnel: [w336] -> w134
            tunnel: w133 -> [w335]
            tunnel: [w335] -> w132
            frame #0 {
              n220 = Wait (ms)(milliseconds to wait=u32 1000) -> ()  [unwired: 1 out]
            }
          }
          n221 = Initialize Array(0.0 ("element"), w168) -> (w166:dbl[])
          n222 = Initialize Array(0.0 ("element"), w293) -> (w165:dbl[])
          n223 = while {
            tunnel: w323 -> [w379]
            tunnel: [w378] -> w193
            shift-right: [w389] -> w174
            shift-left: w132 -> [w383]
            shift-right: [w385] -> w175
            shift-left: w134 -> [w384]
            shift-right: [w414] -> w290
            shift-left: w165 -> [w397]
            shift-right: [w415] -> w324
            shift-left: w166 -> [w395]
            shift-right: [w391] -> w151
            shift-left: w163 -> [w396]
            shift-right: [w393] -> w291
            shift-left: w165 -> [w392]
            tunnel: 0 -> [w390]
            tunnel: w156 -> [w374]
            tunnel: w155 -> [w375]
            tunnel: [w373] -> w154
            tunnel: [w372] -> w153
            tunnel: w149 -> [w371]
            tunnel: w141 -> [_]
            tunnel: w136 -> [w363]
            stop <- w398 stop-if-true
            w355 = TRUE ("element")
            n224 = flat-sequence {
              tunnel: w384 -> [w481]
              tunnel: [w478] -> w380
              tunnel: [w477] -> w381
              tunnel: [w485] -> w370
              tunnel: w383 -> [w480]
              tunnel: w375 -> [w476]
              tunnel: w374 -> [w475]
              tunnel: [w474] -> w373
              tunnel: [w473] -> w372
              tunnel: w371 -> [w472]
              tunnel: w363 -> [w459]
              frame #0 {
                # "To synch DAQ and scope acquisitions"
                n225 = local read "Averages on scope"() -> (w484:i32)
                n226 = local read "DAQ LED line"() -> (w463:string)
                n227 = Equal?(x=w484, y=1.0) -> (x = y?=w482:bool)
                n228 = call "Initiate.vi"("error in (no error)"=w480, "VISA resource name"=w481) -> ("error out"=w469:errorcluster, "VISA resource name out"=w471:refnum<visa-resource-name>)  [unwired: 8 in]
                n229 = Multiply(x="LED on (s)", y=1000.0) -> (x*y=w464:dbl)
                n230 = case shown="True" w482 {
                  tunnel: [w525 w531] -> w485
                  tunnel: w476 -> [w524 w530]
                  tunnel: w475 -> [w523 w529]
                  tunnel: [w521 w528] -> w474
                  tunnel: [w520 w527] -> w473
                  tunnel: w472 -> [_ w526]
                  frame True {
                    # "No averages on scope, acquire one shot"
                    n231 = call-poly <vilib>:"DAQmx Read.vi"("task/channels in"=w524, "number of samples per channel"=-1, "timeout"=300.0, "error in"=w523) -> ("task out"=w521:refnum<k21>, "data"=w525:waveform(dbl), "error out"=w520:errorcluster)  [unwired: 9 in]
                  }
                  frame False {
                    # "Averaging on scope, acquire multiple shots."
                    n232 = while {
                      shift-right: [w545] -> w531
                      shift-left: w526 -> [w544]
                      tunnel: w530 -> [w538]
                      tunnel: w529 -> [w537]
                      tunnel: [w534] -> w528
                      tunnel: [w533] -> w527
                      i -> [w541]
                      stop <- w543 stop-if-true
                      n233 = call-poly <vilib>:"DAQmx Read.vi"("task/channels in"=w538, "number of samples per channel"=-1, "timeout"=20.0, "error in"=w537) -> ("task out"=w534:refnum<k21>, "data"=w539:waveform(dbl), "error out"=w533:errorcluster)  [unwired: 9 in]
                      n234 = local read "Averages on scope"() -> (w542:i32)
                      n235 = Add(x=w541, y=1) -> (x+y=w535:i32)
                      "DAQ Loop" <- w535
                      n236 = Greater Or Equal?(x=w535, y=w542) -> (x >= y?=w543:bool)
                      n237 = Add(1:w544, 2:w539) -> (0:w545:waveform(dbl))  [unwired: 1 in, 1 out]
                    }
                  }
                }
                n238 = Multiply(x="LED off (s)", y=1000.0) -> (x*y=w460:dbl)
                n239 = case shown="True" "PIA Mode" {
                  tunnel: w471 -> [w487 w501]
                  tunnel: [w487 w495] -> w470
                  tunnel: w469 -> [w486 w500]
                  tunnel: [w486 w496] -> w468
                  tunnel: w464 -> [_ w499]
                  tunnel: w463 -> [_ w494]
                  tunnel: w460 -> [_ w493]
                  tunnel: w459 -> [_ w488]
                  frame False {
                  }
                  frame True {
                    n240 = flat-sequence {
                      tunnel: w494 -> [w510]
                      tunnel: w500 -> [w511]
                      tunnel: w501 -> [w512]
                      tunnel: [w512] -> w492
                      tunnel: [w511] -> w491
                      tunnel: [w510] -> w490
                      tunnel: [w509] -> w489
                      tunnel: w488 -> [w508]
                      tunnel: [w517] -> w498
                      tunnel: [w518] -> w497
                      tunnel: [w516] -> _
                      tunnel: w499 -> [w515]
                      tunnel: w492 -> [w517]
                      tunnel: w491 -> [w518]
                      tunnel: w490 -> [w514]
                      tunnel: w489 -> [_]
                      frame #0 {
                        n241 = Wait (ms)(milliseconds to wait=w508) -> (millisecond timer value=w509:u32)
                      }
                      frame #1 {
                        n242 = call "RG DAQ control for PIA.vi"("lines"=w514, "Initial value"=TRUE) -> ()  [unwired: 10 in]
                        n243 = Wait (ms)(milliseconds to wait=w515) -> (millisecond timer value=w516:u32)
                      }
                    }
                    n244 = flat-sequence {
                      tunnel: w498 -> [w507]
                      tunnel: [w507] -> w495
                      tunnel: [w506] -> _
                      tunnel: w493 -> [w505]
                      tunnel: w494 -> [w504]
                      tunnel: w497 -> [w502]
                      tunnel: [w502] -> w496
                      frame #0 {
                        n245 = call "RG DAQ control for PIA.vi"("lines"=w504, "Initial value"=FALSE) -> ()  [unwired: 10 in]
                        n246 = Wait (ms)(milliseconds to wait=w505) -> (millisecond timer value=w506:u32)
                      }
                    }
                  }
                }
                n247 = VISA Write(VISA resource name=w470, write buffer="*WAI", error in (no error)=w468) -> (VISA resource name out=w478:refnum<visa-resource-name>, error out=w477:errorcluster)  [unwired: 1 out]
              }
            }
            n248 = local read "Scope Timeout (ms)"() -> (w382:u32)
            n249 = local read "DAQ Number of Samples"() -> (w367:dbl)
            n250 = call "RG Fetch Waveforms from scope.vi"("error in (no error)"=w381, "Maximum Time (10000ms)"=w382, "Channels"=w379, "VISA resource name"=w380) -> ("error out"=w376:errorcluster, "Waveform Data"=w378:waveform(dbl)[], "VISA resource name out"=w377:refnum<visa-resource-name>)  [unwired: 5 in]
            n251 = Unbundle By Name(w376) -> ("status"=w388:bool)
            n252 = local read "Scope average\nnumber of points"() -> (w411:dbl)
            n253 = local read "DAQ rate"() -> (w364:i32)
            n254 = Multiply(x=w367, y=-0.1) -> (x*y=w365:dbl)
            n255 = local read "DAQ average number of points"() -> (w402:dbl)
            n256 = Divide(x=w365, y=w364) -> (x/y=w368:dbl)
            n257 = Split Signals(w378) -> (w409:dynamicdata, w408:dynamicdata)  [unwired: 2 in]
            n258 = To Time Stamp(1:w368) -> (0:w369:timestamp)
            n259 = Unbundle By Name(w370) -> ("Y"=w403:dbl[])
            n260 = call "Convert from Dynamic Data2"("Dynamic Data Type"=w409) -> ("Array"=w387:dbl[])  [unwired: 3 in]
            n261 = call "Convert from Dynamic Data3"("Dynamic Data Type"=w408) -> ("Array"=w407:dbl[])  [unwired: 3 in]
            n262 = Empty Array?(array=w387) -> (empty?=w386:bool)
            n263 = Bundle By Name(cluster=w370, "t0"=w369) -> (w356:waveform(dbl))
            n264 = case shown="False" "Inspect Traces" {
              tunnel: [TRUE w419] -> w357
              tunnel: w356 -> [w416 w418]
              frame False {
                n265 = local write "DAQ Live Data"(w416) -> ()
              }
              frame True {
                n266 = call "User trace inspection"() -> ("yes - keep it."=w419:bool)  [unwired: 18 in, 1 out]
                "DAQ Live Data" <- w418
              }
            }
            n267 = call-poly <vilib>:"Decimate (single shot).vi"("averaging"=TRUE, "decimating factor"=w402, "X"=w403) -> ("Decimated Array"=w394:dbl[])  [unwired: 7 in, 1 out]
            n268 = Not Or(1:w386, 2:w388) -> (0:w362:bool)
            n269 = call-poly <vilib>:"Decimate (single shot).vi"("averaging"=TRUE, "decimating factor"=w411, "X"=w387) -> ("Decimated Array"=w399:dbl[])  [unwired: 7 in, 1 out]
            n270 = call-poly <vilib>:"Decimate (single shot).vi"("averaging"=TRUE, "decimating factor"=w411, "X"=w407) -> ("Decimated Array"=w400:dbl[])  [unwired: 7 in, 1 out]
            n271 = Build Array(w355, w357, w355, w362) -> (w361:bool[])
            n272 = Search 1D Array(1D array=w361, element=FALSE) -> (index of element=w359:i32)  [unwired: 1 in]
            n273 = case shown="3" w359 {
              tunnel: [w425 w439 w451] -> w415
              tunnel: [w424 w438 w450] -> w414
              tunnel: [w422 w429 w445] -> w413
              tunnel: w400 -> [_ w437 _]
              tunnel: w399 -> [_ w436 _]
              tunnel: w397 -> [w424 w435 w450]
              tunnel: w396 -> [w422 w434 w445]
              tunnel: w395 -> [w425 w433 w451]
              tunnel: w394 -> [_ w432 _]
              tunnel: [w423 w431 w449] -> w393
              tunnel: w392 -> [w423 w430 w449]
              tunnel: [w422 w429 w445] -> w391
              tunnel: w390 -> [_ _ w447]
              tunnel: w376 -> [w420 w428 w443]
              tunnel: [w420 w428 w441] -> w389
              tunnel: w377 -> [w421 w427 w444]
              tunnel: [w421 w427 w440] -> w385
              frame 1 {
                # "User Rejects Trace"
              }
              frame 2, Default {
                # "No errors"
                n274 = local read "Averages on scope"() -> (w426:i32)
                n275 = Add(x=w426, y=w434) -> (x+y=w429:i32)
                "Readout Counter" <- w429
                n276 = Add(x=w432, y=w433) -> (x+y=w439:dbl[])
                n277 = Add(x=w435, y=w436) -> (x+y=w438:dbl[])
                n278 = Add(x=w437, y=w430) -> (x+y=w431:dbl[])
              }
              frame 3 {
                # "Scope Error Detected"
                n279 = flat-sequence {
                  tunnel: w444 -> [w452]
                  tunnel: w443 -> [w453]
                  tunnel: [w452] -> w442
                  tunnel: w442 -> [w458]
                  tunnel: [w455] -> w441
                  tunnel: [w454] -> w440
                  frame #0 {
                    n280 = call "Close.vi"("error in (no error)"=w453, "VISA resource name"=w452) -> ()  [unwired: 9 in, 1 out]
                  }
                  frame #1 {
                    w457 = FALSE ("ID Query (True)")
                    n281 = call "Initialize.vi"("error in (no error)"=errorcluster {"status"=FALSE, "code"=0, "source"=""}, "Reset (True)"=w457, "ID Query (True)"=w457, "VISA resource name"=w458) -> ("error out"=w455:errorcluster, "VISA resource name out"=w454:refnum<visa-resource-name>)  [unwired: 6 in]
                  }
                }
                n282 = Add(x=w447, y=1.0) -> (x+y=→"Scope Error Counter":dbl)
              }
            }
            n283 = local read "Number of Averages"() -> (w406:i32)
            n284 = Greater Or Equal?(x=w413, y=w406) -> (x >= y?=w405:bool)
            n285 = Or(x=w405, y="Stop Measurement") -> (x .or. y?=w398:bool)
          }
          n286 = call-poly <vilib>:"Index Waveform Array.vi"("index"=0, "waveform array"=w193) -> ("waveform"=w191:waveform(dbl))  [unwired: 8 in, 1 out]
          n287 = Unbundle By Name(w191) -> ("t0"=w173:timestamp, "dt"=w172:dbl)
          n288 = local read "Record Length"() -> (w187:u32)
          n289 = To Double Precision Float(number=w173) -> (double precision float=w190:dbl)
          n290 = Multiply(x=w187, y=1000.0) -> (x*y=w189:dbl)
          n291 = local read "Scope average\nnumber of points"() -> (w184:dbl)
          n292 = for {
            N: w189 -> [_]
            tunnel: w190 -> [w557]
            tunnel: w172 -> [w555]
            tunnel: [w553] -> w186 mode=indexing
            i -> [w556]
            n293 = Multiply(x=w555, y=w556) -> (x*y=w554:dbl)
            n294 = Add(x=w557, y=w554) -> (x+y=w553:dbl)
          }
          n295 = call-poly <vilib>:"Decimate (single shot).vi"("averaging"=TRUE, "decimating factor"=w184, "X"=w186) -> ("Decimated Array"=w104:dbl[])  [unwired: 7 in, 1 out]
          "Scope time axis" <- w104
          n296 = call <vilib>:"DAQmx Clear Task.vi"("task in"=w154, "error in"=w153) -> ()  [unwired: 13 in, 1 out]
          n297 = local read "Averages on scope"() -> (w152:i32)
          n298 = Divide(x=w151, y=w152) -> (x/y=w150:dbl)
          n299 = Divide(x=w291, y=w150) -> (x/y=w333:dbl[])
          n300 = Divide(x=w290, y=w150) -> (x/y=w226:dbl[])
          n301 = local read "DAQ final number of points"() -> (w148:dbl)
          n302 = Bundle By Name("Y"=w333, "t0"=w173, "dt"=w172) -> (→"Scope Average Channel2":waveform(dbl))  [unwired: 1 in]
          n303 = Bundle By Name("Y"=w226, "t0"=w173, "dt"=w172) -> (→"Scope Average Channel1":waveform(dbl))  [unwired: 1 in]
          n304 = local read "DAQ average number of points"() -> (w294:dbl)
          n305 = Divide(x=w324, y=w151) -> (x/y=w194:dbl[])
          n306 = local read "DAQ dt"() -> (w295:dbl)
          n307 = Multiply(x=w148, y=-0.1) -> (x*y=w145:dbl)
          n308 = Multiply(x=w295, y=w294) -> (x*y=w146:dbl)
          n309 = Multiply(x=w145, y=w146) -> (x*y=w143:dbl)
          n310 = To Time Stamp(1:w143) -> (0:w144:timestamp)
          n311 = local read "DAQ final number of points"() -> (w302:dbl)
          n312 = Bundle By Name("Y"=w194, "t0"=w144, "dt"=w146) -> (→"DAQ Average Data":waveform(dbl))  [unwired: 1 in]
          n313 = Multiply(x=w302, y=0.075) -> (x*y=w297:dbl)
          n314 = Round To Nearest(number=w297) -> (nearest integer value=w296:dbl)
          n315 = Array Subset(array=w194, index=0, length=w296) -> (w318:dbl[])
          n316 = local read "Amplification Factor"() -> (w316:dbl)
          n317 = Add Array Elements(numeric array=w318) -> (sum=w317:dbl)
          n318 = Divide(x=w317, y=w296) -> (x/y=w170:dbl)
          n319 = Multiply(x=w170, y=w316) -> (x*y=w171:dbl)
          n320 = local write "Background level (on Amp)"(w171) -> ()
          n321 = local write "Background level (V)"(w170) -> ()
          n322 = local read "DAQ Number of Samples"() -> (w177:dbl)
          n323 = for {
            N: w177 -> [_]
            tunnel: [w547] -> w178 mode=indexing
            i -> [w552]
            n324 = local read "DAQ Number of Samples"() -> (w551:dbl)
            n325 = Divide(x=w551, y=10.0) -> (x/y=w549:dbl)
            n326 = local read "DAQ dt"() -> (w546:dbl)
            n327 = Subtract(x=w552, y=w549) -> (x-y=w548:dbl)
            n328 = Multiply(x=w548, y=w546) -> (x*y=w547:dbl)
          }
          n329 = local read "DAQ average number of points"() -> (w180:dbl)
          n330 = Number To Decimal String(number=w206, width (-)=i16 3) -> (decimal integer string=w205:string)
          n331 = call-poly <vilib>:"Decimate (single shot).vi"("averaging"=TRUE, "decimating factor"=w180, "X"=w178) -> ("Decimated Array"=w176:dbl[])  [unwired: 7 in, 1 out]
          n332 = Concatenate Strings(w205, "nm Scope CH2 (raw data).txt") -> (w218:string)
          n333 = global read "global tas.vi" "Root Path"() -> (w282:path)
          n334 = Build Array(w176, w194) -> (w283:dbl[][])
          n335 = Build Array(w104, w226) -> (w273:dbl[][])
          n336 = global read "global tas.vi" "Root Path"() -> (w277:path)
          n337 = Concatenate Strings(w205, "nm DAQ (raw data).txt") -> (w221:string)
          n338 = global read "global tas.vi" "Root Path"() -> (w204:path)
          n339 = Build Array(w104, w333) -> (w278:dbl[][])
          n340 = Concatenate Strings(w205, "nm Scope CH1 (raw data).txt") -> (w216:string)
          n341 = Build Path(base path=w282, name or relative path=w221) -> (appended path=w281:path)
          n342 = Build Path(base path=w277, name or relative path=w218) -> (appended path=w276:path)
          n343 = Build Path(base path=w204, name or relative path=w216) -> (appended path=w272:path)
          n344 = call-poly <vilib>:"Write To Spreadsheet File.vi"("transpose? (no:F)"=TRUE, "format (%.3f)"="%.9f", "2D data"=w283, "file path (dialog if empty)"=w281) -> ()  [unwired: 4 in, 1 out]
          n345 = call-poly <vilib>:"Write To Spreadsheet File.vi"("transpose? (no:F)"=TRUE, "format (%.3f)"="%.9f", "2D data"=w273, "file path (dialog if empty)"=w272) -> ()  [unwired: 4 in, 1 out]
          n346 = call-poly <vilib>:"Write To Spreadsheet File.vi"("transpose? (no:F)"=TRUE, "format (%.3f)"="%.9f", "2D data"=w278, "file path (dialog if empty)"=w276) -> ()  [unwired: 4 in, 1 out]
          n347 = flat-sequence {
            tunnel: w205 -> [w691]
            tunnel: w204 -> [w690]
            tunnel: w169 -> [_]
            frame #0 {
              # "Write parameters file after values have been calculated."
              n348 = Build Array("Number of Averages", "Scope acq. type", "Number of averages on scope", "Scope average number of points", "Scope timebase (s)", "Scope CH1 vertical scale per div (V)", "Scope CH2 vertical scale per div (V)", "Background level on amp (V)", "DAQ sampling rate (Hz)", "DAQ average number of points", "Background level on DAQ (V)", "Amplification factor", "100% Reflection Reference Signal (V)" ("element"), "Output calculation Method" ("element")) -> (w715:string[])
              n349 = Concatenate Strings(w691, "nm Parameters.txt") -> (w693:string)
              n350 = local read "Scope Timebase (per div)"() -> (w707:dbl)
              n351 = local read "Averages on scope"() -> (w706:i32)
              n352 = local read "DAQ rate"() -> (w711:i32)
              n353 = local read "Acquisition Type"() -> (w724:u16)
              n354 = Build Path(base path=w690, name or relative path=w693) -> (appended path=w717:path)
              n355 = local read "Scope average\nnumber of points"() -> (w705:dbl)
              n356 = local read "Vertical Range CH TAS (10.0 V)"() -> (w708:dbl)
              n357 = local read "Vertical Range TPC (10.0 V)"() -> (w709:dbl)
              n358 = local read "Background level (on Amp)"() -> (w710:dbl)
              n359 = local read "DAQ average number of points"() -> (w712:dbl)
              n360 = local read "Background level (V)"() -> (w713:dbl)
              n361 = local read "Amplification Factor"() -> (w714:dbl)
              n362 = local read "100% Reflectance Standard (V)"() -> (w726:dbl)
              n363 = local read "Calculate Output Method"() -> (w728:T1)
              n364 = local read "Readout Counter"() -> (w722:i32)
              n365 = Build Array(w722, w724, w706, w705, w707, w708, w709, w710, w711, w712, w713, w714, w726, w728) -> (w716:dbl[])
              n366 = Number To Fractional String(number=w716) -> (F-format string=w692:string[])  [unwired: 3 in]
              n367 = Build Array(w715, w692) -> (w718:string[][])
              n368 = Array To Spreadsheet String(array=w718, 3:"%s" ("format string")) -> (spreadsheet string=w720:string)  [unwired: 1 in]
              n369 = Write to Text File(file (use dialog)=w717, text=w720) -> ()  [unwired: 2 in, 3 out]
            }
          }
          n370 = local read "Calculate Output Method"() -> (w238:T1)
          n371 = local read "TPC Multiplication factor"() -> (w258:dbl)
          n372 = case shown="\"Reflectance\"" w238 {
            tunnel: w194 -> [w759 w764 w782]
            tunnel: [w758 w762 w774] -> w109
            tunnel: w170 -> [w757 w761 w765]
            frame "Transmission" {
              # "Background level on DAQ"
              # "Calculate output as: deltaOD = log(T/T')"
              n373 = Divide(x=w757, y=w759) -> (x/y=w760:dbl[])
              n374 = Logarithm Base 10(1:w760) -> (0:w758:dbl[])
            }
            frame "Reflectance" {
              # "Calculate output as: Transient abs. = 1 - RT = (Rbkg - R(t)) / Rbkg"
              n375 = Subtract(x=w761, y=w764) -> (x-y=w763:dbl[])
              n376 = Divide(x=w763, y=w761) -> (x/y=w762:dbl[])
            }
            frame "Kubelka-Munk" {
              # "Calculate output from\nKM = (1-Rrelative)^2/(2*Rrelative)"
              n377 = local read "100% Reflectance Standard (V)"() -> (w781:dbl)
              n378 = Divide(x=w782, y=w781) -> (x/y=w767:dbl[])
              n379 = Subtract(x=1.0, y=w767) -> (x-y=w769:dbl[])
              n380 = Divide(x=w765, y=w781) -> (x/y=w776:dbl)
              n381 = Square(x=w769) -> (x^2=w770:dbl[])
              n382 = Subtract(x=1.0, y=w776) -> (x-y=w779:dbl)
              n383 = Multiply(x=w767, y=2.0) -> (x*y=w771:dbl[])
              n384 = Square(x=w779) -> (x^2=w778:dbl)
              n385 = Divide(x=w770, y=w771) -> (x/y=w766:dbl[])
              n386 = Multiply(x=w776, y=2.0) -> (x*y=w777:dbl)
              n387 = Divide(x=w778, y=w777) -> (x/y=w773:dbl)
              n388 = Subtract(x=w766, y=w773) -> (x-y=w774:dbl[])
            }
          }
          n389 = local read "DAQ average number of points"() -> (w231:dbl)
          n390 = local read "DAQ final number of points"() -> (w242:dbl)
          n391 = Multiply(x=w333, y=w258) -> (x*y=w125:dbl[])
          n392 = local read "DAQ dt"() -> (w232:dbl)
          n393 = local read "Scope pretrigger points"() -> (w246:dbl)
          n394 = Multiply(x=w232, y=w231) -> (x*y=w233:dbl)
          n395 = Divide(x=w242, y=-10.0) -> (x/y=w241:dbl)
          n396 = Multiply(x=w241, y=w233) -> (x*y=w240:dbl)
          n397 = To Time Stamp(1:w240) -> (0:w239:timestamp)
          n398 = Multiply(x=w246, y=0.75) -> (x*y=w245:dbl)
          n399 = Bundle By Name("Y"=w125, "t0"=w173, "dt"=w172) -> (→"Scope CH2 data (final)":waveform(dbl))  [unwired: 1 in]
          n400 = Array Subset(array=w226, index=0, length=w245) -> (w249:dbl[])
          n401 = Add Array Elements(numeric array=w249) -> (sum=w250:dbl)
          n402 = Divide(x=w250, y=w245) -> (x/y=w251:dbl)
          n403 = Subtract(x=w226, y=w251) -> (x-y=w237:dbl[])
          n404 = local read "Calculate Output Method"() -> (w234:T1)
          n405 = Bundle By Name("Y"=w109, "t0"=w239, "dt"=w233) -> (→"DAQ DOD data (final)":waveform(dbl))  [unwired: 1 in]
          n406 = Add(x=w237, y=w171) -> (x+y=w236:dbl[])
          n407 = case shown="\"Reflectance\"" w234 {
            tunnel: w236 -> [w730 w736 w755]
            tunnel: [w729 w733 w748] -> w235
            frame "Transmission" {
              # "Calculate output as: deltaOD = log(T/T')"
              n408 = local read "Background level (on Amp)"() -> (w731:dbl)
              n409 = Divide(x=w731, y=w730) -> (x/y=w732:dbl[])
              n410 = Logarithm Base 10(1:w732) -> (0:w729:dbl[])
            }
            frame "Reflectance" {
              # "Calculate output as: Transient abs. = 1 - RT = (Rbkg - R(t)) / Rbkg"
              n411 = local read "Background level (on Amp)"() -> (w735:dbl)
              n412 = Subtract(x=w735, y=w736) -> (x-y=w734:dbl[])
              n413 = Divide(x=w734, y=w735) -> (x/y=w733:dbl[])
            }
            frame "Kubelka-Munk" {
              # "Calculate output from\nKM = (1-Rrelative)^2/(2*Rrelative)"
              n414 = local read "100% Reflectance Standard (V)"() -> (w738:dbl)
              n415 = local read "Amplification Factor"() -> (w739:dbl)
              n416 = local read "Background level (on Amp)"() -> (w756:dbl)
              n417 = Multiply(x=w738, y=w739) -> (x*y=w737:dbl)
              n418 = Divide(x=w755, y=w737) -> (x/y=w741:dbl[])
              n419 = Subtract(x=1.0, y=w741) -> (x-y=w743:dbl[])
              n420 = Divide(x=w756, y=w737) -> (x/y=w750:dbl)
              n421 = Square(x=w743) -> (x^2=w744:dbl[])
              n422 = Subtract(x=1.0, y=w750) -> (x-y=w753:dbl)
              n423 = Multiply(x=w741, y=2.0) -> (x*y=w745:dbl[])
              n424 = Square(x=w753) -> (x^2=w752:dbl)
              n425 = Divide(x=w744, y=w745) -> (x/y=w740:dbl[])
              n426 = Multiply(x=w750, y=2.0) -> (x*y=w751:dbl)
              n427 = Divide(x=w752, y=w751) -> (x/y=w747:dbl)
              n428 = Subtract(x=w740, y=w747) -> (x-y=w748:dbl[])
            }
          }
          n429 = local read "DAQ Number of Samples"() -> (w247:dbl)
          n430 = for {
            N: w247 -> [_]
            tunnel: [w784] -> w183 mode=indexing
            i -> [w789]
            n431 = local read "DAQ Number of Samples"() -> (w788:dbl)
            n432 = Divide(x=w788, y=10.0) -> (x/y=w786:dbl)
            n433 = local read "DAQ dt"() -> (w783:dbl)
            n434 = Subtract(x=w789, y=w786) -> (x-y=w785:dbl)
            n435 = Multiply(x=w785, y=w783) -> (x*y=w784:dbl)
          }
          n436 = Number To Decimal String(number=w206, width (-)=i16 3) -> (decimal integer string=w128:string)
          n437 = local read "DAQ average number of points"() -> (w181:dbl)
          n438 = Concatenate Strings(w128, "nm Scope CH1 (final A).txt") -> (w209:string)
          n439 = Build Array(w104, w125) -> (w264:dbl[][])
          n440 = global read "global tas.vi" "Root Path"() -> (w255:path)
          n441 = Concatenate Strings(w128, "nm Scope CH2 (final).txt") -> (w211:string)
          n442 = global read "global tas.vi" "Root Path"() -> (w263:path)
          n443 = Build Path(base path=w255, name or relative path=w209) -> (appended path=w254:path)
          n444 = Array Size(array=w104) -> (size(s)=w123:i32)
          n445 = Build Path(base path=w263, name or relative path=w211) -> (appended path=w262:path)
          n446 = call-poly <vilib>:"Decimate (single shot).vi"("averaging"=TRUE, "decimating factor"=w181, "X"=w183) -> ("Decimated Array"=w107:dbl[])  [unwired: 7 in, 1 out]
          n447 = Multiply(x=w123, y=0.95) -> (x*y=w122:dbl)
          n448 = call-poly <vilib>:"Write To Spreadsheet File.vi"("transpose? (no:F)"=TRUE, "format (%.3f)"="%.9f", "2D data"=w264, "file path (dialog if empty)"=w262) -> ()  [unwired: 4 in, 1 out]
          n449 = Bundle By Name("Y"=w235, "t0"=w173, "dt"=w172) -> (w228:waveform(dbl))  [unwired: 1 in]
          "Scope CH1 DOD data (A final)" <- w228
          n450 = Build Array(w107, w109) -> (w257:dbl[][])
          n451 = global read "global tas.vi" "Root Path"() -> (w266:path)
          n452 = Build Array(w104, w235) -> (w256:dbl[][])
          n453 = Array Subset(array=w104, index=w122) -> (w120:dbl[])  [unwired: 1 in]
          n454 = call-poly <vilib>:"Write To Spreadsheet File.vi"("transpose? (no:F)"=TRUE, "format (%.3f)"="%.9f", "2D data"=w256, "file path (dialog if empty)"=w254) -> ("new file path (Not A Path if cancelled)"=w169:path)  [unwired: 4 in]
          n455 = Concatenate Strings(w128, "nm DAQ DOD (final).txt") -> (w213:string)
          n456 = local read "Trace B ?"() -> (w229:bool)
          n457 = Array Max & Min(array=w120) -> (max value=w119:dbl, min value=w118:dbl)  [unwired: 2 out]
          n458 = Build Path(base path=w266, name or relative path=w213) -> (appended path=w267:path)
          n459 = Threshold 1D Array(2:w118, 3:w107) -> (0:w117:dbl)  [unwired: 1 in]
          n460 = Threshold 1D Array(2:w119, 3:w107) -> (0:w106:dbl)  [unwired: 1 in]
          n461 = Subtract(x=w106, y=w117) -> (x-y=w116:dbl)
          n462 = case shown="True" w229 {
            tunnel: w228 -> [_ _]
            tunnel: [u32 0 ("millisecond timer value") w914] -> w227
            tunnel: w151 -> [_ _]
            frame False {
            }
            frame True {
              w927 = u32 10000  # timeout (10sec)
              # "Note:Closing the serial port allows it to be used by other applications without quitting LabVIEW."
              # "Close session to port."
              # "Configure Serial port (baud rate, data bits, parity, stop bits and flow control)."
              # "Write bytes to port."
              n463 = Wait (ms)(milliseconds to wait=u32 20000) -> (millisecond timer value=w914:u32)
              n464 = local read "Shutter VISA resource name"() -> (w921:refnum<visa-resource-name>)
              n465 = local read "Shutter data bits"() -> (w918:u16)
              n466 = local read "Shutter baud rate"() -> (w920:u32)
              n467 = local read "Shutter parity"() -> (w919:u16)
              n468 = local read "Shutter flow control"() -> (w917:u16)
              n469 = local read "Shutter stop bits"() -> (w916:u16)
              n470 = local read "Shutter open string"() -> (w913:string)
              n471 = call-poly "VISA Configure Serial Port"("VISA resource name"=w921, "timeout (10sec)"=w927, "baud rate (9600)"=w920, "data bits (8)"=w918, "parity (0:none)"=w919, "stop bits (10: 1 bit)"=w916, "flow control (0:none)"=w917) -> ("VISA resource name out"=w926:refnum<visa-resource-name>, "error out"=w925:errorcluster)  [unwired: 2 in, 5 out]
              n472 = VISA Write(VISA resource name=w926, write buffer=w913, error in (no error)=w925) -> (VISA resource name out=w923:refnum<visa-resource-name>, error out=w922:errorcluster)  [unwired: 1 out]
              n473 = VISA Close(VISA resource name=w923, error in (no error)=w922) -> (error out=w924:errorcluster)
              n474 = call <vilib>:"Simple Error Handler.vi"("error in (no error)"=w924) -> ()  [unwired: 1 in, 8 out]
            }
          }
          n475 = Array Subset(array=w109, index=w117, length=w116) -> (w115:dbl[])
          n476 = call-poly <vilib>:"Write To Spreadsheet File.vi"("transpose? (no:F)"=TRUE, "format (%.3f)"="%.9f", "2D data"=w257, "file path (dialog if empty)"=w267) -> ()  [unwired: 4 in, 1 out]
          n477 = call-poly <vilib>:"Mean.vi"("X"=w115) -> ("mean"=w112:dbl)  [unwired: 1 out]
          n478 = case shown="False" w229 {
            tunnel: w237 -> [_ w844]
            tunnel: w227 -> [_ _]
            tunnel: [w794 w804] -> w207
            tunnel: w206 -> [_ w803]
            tunnel: w104 -> [_ w802]
            tunnel: w175 -> [w792 w801]
            tunnel: w174 -> [w791 w800]
            tunnel: [dbl[] [] w796] -> w100
            frame False {
              n479 = call "Close.vi"("error in (no error)"=w791, "VISA resource name"=w792) -> ("error out"=w793:errorcluster)  [unwired: 9 in]
              n480 = call <vilib>:"Simple Error Handler.vi"("error in (no error)"=w793) -> ()  [unwired: 4 in, 5 out]
              n481 = Wait (ms)(milliseconds to wait=u32 1) -> (millisecond timer value=w794:u32)
            }
            frame True {
              # "Scope time axis"
              # "Current wavelength"
              n482 = local read "Final number of\nscope points"() -> (w817:dbl)
              n483 = Initialize Array(0.0 ("element"), w817) -> (w818:dbl[])
              n484 = while {
                tunnel: w801 -> [w854]
                tunnel: [w863] -> w851
                tunnel: w800 -> [w853]
                tunnel: [w862] -> w852
                shift-right: [w881] -> w820
                shift-left: w818 -> [w880]
                shift-right: [w864] -> w799
                shift-left: 0 -> [w865]
                stop <- w877 stop-if-true
                n485 = local read "Channel TAS (0: Channel 1)"() -> (w859:u16)
                n486 = local read "Scope Timeout (ms)"() -> (w860:u32)
                n487 = call "RG Read (Single Waveform) change OPC for WAIT.vi"("error in (no error)"=w853, "Maximum Time (10000ms)"=w860, "Channel (0: Channel 1)"=w859, "VISA resource name"=w854) -> ("error out"=w856:errorcluster, "Waveform Graph"=w858:waveform(dbl), "VISA resource name out"=w857:refnum<visa-resource-name>)  [unwired: 5 in]
                "B trace (Channel1)" <- w858
                n488 = local read "Scope average\nnumber of points"() -> (w882:dbl)
                n489 = Unbundle By Name(w858) -> ("Y"=w875:dbl[])
                n490 = local read "Final number of\nscope points"() -> (w874:dbl)
                n491 = local read "Averages on scope"() -> (w855:i32)
                n492 = call-poly <vilib>:"Decimate (single shot).vi"("averaging"=TRUE, "decimating factor"=w882, "X"=w875) -> ("Decimated Array"=w871:dbl[])  [unwired: 7 in, 1 out]
                n493 = Array Size(array=w871) -> (size(s)=w870:i32)
                n494 = Initialize Array(0.0 ("element"), w874) -> (w872:dbl[])
                n495 = Equal To 0?(x=w870) -> (x = 0?=w867:bool)
                n496 = Select(t=0.0, s=w867, f=w855) -> (s? t:f=w866:dbl)
                n497 = Add(x=w865, y=w866) -> (x+y=w864:dbl)
                "Btrace Readout Counter" <- w864
                n498 = local read "Number of Averages"() -> (w879:i32)
                n499 = Select(t=w872, s=w867, f=w871) -> (s? t:f=w869:dbl[])
                n500 = VISA Write(VISA resource name=w857, write buffer="*WAI", error in (no error)=w856) -> (VISA resource name out=w863:refnum<visa-resource-name>, error out=w862:errorcluster)  [unwired: 1 out]
                n501 = Add(x=w880, y=w869) -> (x+y=w881:dbl[])
                n502 = Greater Or Equal?(x=w864, y=w879) -> (x >= y?=w878:bool)
                n503 = Or(x=w878, y="Stop Btrace Measurement") -> (x .or. y?=w877:bool)
              }
              n504 = Number To Decimal String(number=w803, width (-)=i16 3) -> (decimal integer string=w806:string)
              n505 = Concatenate Strings(w806, "nm Scope CH1 B trace (raw data).txt") -> (w810:string)
              n506 = global read "global tas.vi" "Root Path"() -> (w822:path)
              n507 = Build Path(base path=w822, name or relative path=w810) -> (appended path=w821:path)
              n508 = local read "Averages on scope"() -> (w798:i32)
              n509 = Divide(x=w799, y=w798) -> (x/y=w797:dbl)
              n510 = local read "Scope pretrigger points"() -> (w828:dbl)
              n511 = Divide(x=w820, y=w797) -> (x/y=w819:dbl[])
              n512 = call "Close.vi"("error in (no error)"=w852, "VISA resource name"=w851) -> ("error out"=w850:errorcluster)  [unwired: 9 in]
              n513 = Build Array(w802, w819) -> (w825:dbl[][])
              n514 = call <vilib>:"Simple Error Handler.vi"("error in (no error)"=w850) -> ()  [unwired: 4 in, 5 out]
              n515 = call-poly <vilib>:"Write To Spreadsheet File.vi"("transpose? (no:F)"=TRUE, "format (%.3f)"="%.9f", "2D data"=w825, "file path (dialog if empty)"=w821) -> ()  [unwired: 4 in, 1 out]
              n516 = Multiply(x=w828, y=0.75) -> (x*y=w829:dbl)
              n517 = Array Subset(array=w819, index=0, length=w829) -> (w847:dbl[])
              n518 = Add Array Elements(numeric array=w847) -> (sum=w848:dbl)
              n519 = Divide(x=w848, y=w829) -> (x/y=w849:dbl)
              n520 = local read "Background level (on Amp)"() -> (w814:dbl)
              n521 = Subtract(x=w819, y=w849) -> (x-y=w845:dbl[])
              n522 = local read "Calculate Output Method"() -> (w826:T1)
              n523 = Subtract(x=w844, y=w845) -> (x-y=w815:dbl[])
              n524 = Add(x=w815, y=w814) -> (x+y=w816:dbl[])
              n525 = case shown="\"Kubelka-Munk\"" w826 {
                tunnel: w816 -> [w885 w891 w910]
                tunnel: [w884 w888 w903] -> w796
                frame "Transmission" {
                  # "Calculate output as: deltaOD = log(T/T')"
                  n526 = local read "Background level (on Amp)"() -> (w886:dbl)
                  n527 = Divide(x=w886, y=w885) -> (x/y=w887:dbl[])
                  n528 = Logarithm Base 10(1:w887) -> (0:w884:dbl[])
                }
                frame "Reflectance" {
                  # "Calculate output as: Transient abs. = 1 - RT = (Rbkg - R(t)) / Rbkg"
                  n529 = local read "Background level (on Amp)"() -> (w890:dbl)
                  n530 = Subtract(x=w890, y=w891) -> (x-y=w889:dbl[])
                  n531 = Divide(x=w889, y=w890) -> (x/y=w888:dbl[])
                }
                frame "Kubelka-Munk" {
                  # "Calculate output from\nKM = (1-Rrelative)^2/(2*Rrelative)"
                  n532 = local read "100% Reflectance Standard (V)"() -> (w893:dbl)
                  n533 = local read "Amplification Factor"() -> (w894:dbl)
                  n534 = local read "Background level (on Amp)"() -> (w911:dbl)
                  n535 = Multiply(x=w893, y=w894) -> (x*y=w892:dbl)
                  n536 = Divide(x=w910, y=w892) -> (x/y=w896:dbl[])
                  n537 = Subtract(x=1.0, y=w896) -> (x-y=w898:dbl[])
                  n538 = Divide(x=w911, y=w892) -> (x/y=w905:dbl)
                  n539 = Square(x=w898) -> (x^2=w899:dbl[])
                  n540 = Subtract(x=1.0, y=w905) -> (x-y=w908:dbl)
                  n541 = Multiply(x=w896, y=2.0) -> (x*y=w900:dbl[])
                  n542 = Square(x=w908) -> (x^2=w907:dbl)
                  n543 = Divide(x=w899, y=w900) -> (x/y=w895:dbl[])
                  n544 = Multiply(x=w905, y=2.0) -> (x*y=w906:dbl)
                  n545 = Divide(x=w907, y=w906) -> (x/y=w902:dbl)
                  n546 = Subtract(x=w895, y=w902) -> (x-y=w903:dbl[])
                }
              }
              n547 = local read "Scope Timebase (per div)"() -> (w831:dbl)
              n548 = local read "Scope pretrigger points"() -> (w830:dbl)
              n549 = Divide(x=w831, y=10.0) -> (x/y=w837:dbl)
              n550 = Divide(x=w831, y=w830) -> (x/y=w832:dbl)
              n551 = Multiply(x=w837, y=-1.0) -> (x*y=w834:dbl)
              n552 = To Time Stamp(1:w834) -> (0:w833:timestamp)
              n553 = global read "global tas.vi" "Root Path"() -> (w839:path)
              n554 = Bundle By Name("Y"=w796, "t0"=w833, "dt"=w832) -> (→"Scope CH1 DOD data (A-B final)":waveform(dbl))  [unwired: 1 in]
              n555 = Concatenate Strings(w806, "nm Scope CH1 (final A-B).txt") -> (w808:string)
              n556 = Build Path(base path=w839, name or relative path=w808) -> (appended path=w840:path)
              n557 = Wait (ms)(milliseconds to wait=u32 1) -> (millisecond timer value=w804:u32)
              n558 = Build Array(w802, w796) -> (w838:dbl[][])
              n559 = call-poly <vilib>:"Write To Spreadsheet File.vi"("transpose? (no:F)"=TRUE, "format (%.3f)"="%.9f", "2D data"=w838, "file path (dialog if empty)"=w840) -> ()  [unwired: 4 in, 1 out]
            }
          }
          n560 = Array Subset(array=w100, index=w122) -> (w121:dbl[])  [unwired: 1 in]
          n561 = call-poly <vilib>:"Mean.vi"("X"=w121) -> ("mean"=w113:dbl)  [unwired: 1 out]
          n562 = Subtract(x=w113, y=w112) -> (x-y=w114:dbl)
          n563 = Subtract(x=w100, y=w114) -> (x-y=w111:dbl[])
          n564 = Array Subset(array=w109, index=w106) -> (w110:dbl[])  [unwired: 1 in]
          n565 = Build Array (concatenate)(w111, w110) -> (w108:dbl[])
          n566 = Array Subset(array=w107, index=w106) -> (w105:dbl[])  [unwired: 1 in]
          n567 = Build Array (concatenate)(w104, w105) -> (w103:dbl[])
          n568 = Build Array(w103, w108) -> (w102:dbl[][])
          n569 = global read "global tas.vi" "Root Path"() -> (w129:path)
          n570 = Concatenate Strings(w128, "nm Stitched Scope-DAQ (final A-B).txt") -> (w130:string)
          n571 = Build Path(base path=w129, name or relative path=w130) -> (appended path=w126:path)
          n572 = call-poly <vilib>:"Write Delimited Spreadsheet.vi"("file path (dialog if empty)"=w126, "format (%.3f)"="%.9f", "2D data"=w102, "transpose? (F)"=TRUE) -> ()  [unwired: 10 in, 2 out]
        }
        n573 = flat-sequence {
          tunnel: w61 -> [_]
          frame #0 {
            w94 = FALSE
            n574 = local write "2b - Spectrum"(w94) -> ()
            n575 = local write "2a - Kinetic"(w94) -> ()
            n576 = One Button Dialog(message="Acquisition complete.") -> ()  [unwired: 1 in, 1 out]
          }
        }
      }
      frame 3 {
        # "Code"
        n577 = case shown="False" w1010 {
          tunnel: w1010 -> [w1087 w1101]
          tunnel: [w1084 w1101] -> w1009
          frame False {
            # "PTI Mono"
            n578 = flat-sequence {
              tunnel: [w1094] -> w1088
              tunnel: w1087 -> [w1094]
              tunnel: w1088 -> [w1100]
              tunnel: [w1100] -> w1085
              tunnel: [w1096] -> w1086
              frame #0 {
                # "Check where mono is"
                n579 = call "UserInputMonoValue.vi"() -> ("Monochromator readout"=w1095:dbl)  [unwired: 17 in, 2 out]
                n580 = local write "Current Wavelength (PTI)"(w1095) -> ()
              }
              frame #1 {
                # "Find out which grating is currently being used"
                n581 = Two Button Dialog(message="Please press the appropriate\nbutton for the grating currently\nselected on the monochromator.", 1:"Visible" ("F button name (\"Cancel\")"), 2:"IR" ("T button name (\"OK\")")) -> (T button?=w1096:bool)
                n582 = local write "Is IR"(w1096) -> ()
              }
            }
            n583 = case shown="True" w1086 {
              tunnel: w1085 -> [w1089 w1090]
              tunnel: [w1089 w1090] -> w1084
              frame False {
              }
              frame True {
                n584 = local read "Current Wavelength (PTI)"() -> (w1093:dbl)
                n585 = Multiply(x=w1093, y=2.0) -> (x*y=w1092:dbl)
                n586 = local write "Current Wavelength (PTI)"(w1092) -> ()
              }
            }
          }
          frame True {
            # "Oriel Mono"
          }
        }
        n587 = case shown="True" w1009 {
          tunnel: [w1012 w1072] -> w1011
          frame False {
            # "PTI Mono"
            n588 = flat-sequence {
              tunnel: [w1016] -> w1013
              tunnel: [w1066] -> _
              tunnel: w1013 -> [w1066]
              tunnel: [w1065] -> w1012
              frame #0 {
                n589 = local read "Is IR"() -> (w1015:bool)
                n590 = call "RG Get User Input Wavelength.vi"() -> ("Go to wavelength"=w1014:i32)  [unwired: 11 in]
                n591 = case shown="True" w1015 {
                  tunnel: [w1019 w1042] -> w1016
                  tunnel: w1014 -> [w1018 w1041]
                  tunnel: w1014 -> [w1017 w1040]
                  frame True {
                    # "Currently in IR"
                    n592 = Greater?(x=w1017, y=1000.0) -> (0:w1020:bool)
                    n593 = case shown="True" w1020 {
                      tunnel: [w1023 w1032] -> w1019
                      tunnel: w1018 -> [w1022 w1031]
                      frame False {
                        n594 = stacked-sequence {
                          seq-local: [_ w1028 _] -> [_ _ w1030]
                          tunnel: [_ _ w1030] -> w1023
                          tunnel: w1022 -> [_ w1028 _]
                          frame #0 {
                            # "switch to visible\nand recal mono"
                            n595 = One Button Dialog(message="Please switch\nto the visible grating\nnow.") -> (true=w1024:bool)  [unwired: 1 in]
                            n596 = case shown="True" w1024 {
                              frame False {
                              }
                              frame True {
                                n597 = call "UserInputMonoValue.vi"() -> ("Monochromator readout"=w1026:dbl)  [unwired: 17 in, 2 out]
                                n598 = local write "Is IR"(FALSE ("Is IR")) -> ()
                                n599 = local write "Current Wavelength (PTI)"(w1026) -> ()
                              }
                            }
                          }
                          frame #1 {
                            # "now in visible, move \nto new wavelength"
                            n600 = local read "Current Wavelength (PTI)"() -> (w1029:dbl)
                            n601 = call "ChazMoveMono.vi"("Move to"=w1028, "Current"=w1029) -> ()  [unwired: 8 in, 2 out]
                          }
                          frame #2 {
                            n602 = local write "Current Wavelength (PTI)"(w1030) -> ()
                          }
                        }
                      }
                      frame True {
                        # "Still in IR"
                        n603 = stacked-sequence {
                          seq-local: [w1033 _] -> [_ w1039]
                          tunnel: [_ w1039] -> w1032
                          tunnel: w1031 -> [w1033 _]
                          frame #0 {
                            n604 = local read "Current Wavelength (PTI)"() -> (w1038:dbl)
                            n605 = Divide(x=w1033, y=2.0) -> (x/y=w1034:dbl)
                            n606 = Divide(x=w1038, y=2.0) -> (x/y=w1035:dbl)
                            n607 = call "ChazMoveMono.vi"("Move to"=w1034, "Current"=w1035) -> ()  [unwired: 8 in, 2 out]
                          }
                          frame #1 {
                            n608 = local write "Current Wavelength (PTI)"(w1039) -> ()
                          }
                        }
                      }
                    }
                  }
                  frame False {
                    # "Currently in Visible"
                    n609 = Greater?(x=w1040, y=1000.0) -> (0:w1043:bool)
                    n610 = case shown="True" w1043 {
                      tunnel: [w1046 w1051] -> w1042
                      tunnel: w1041 -> [w1045 w1050]
                      frame False {
                        # "Still in Visible"
                        n611 = stacked-sequence {
                          seq-local: [w1047 _] -> [_ w1049]
                          tunnel: [_ w1049] -> w1046
                          tunnel: w1045 -> [w1047 _]
                          frame #0 {
                            n612 = local read "Current Wavelength (PTI)"() -> (w1048:dbl)
                            n613 = call "ChazMoveMono.vi"("Move to"=w1047, "Current"=w1048) -> ()  [unwired: 8 in, 2 out]
                          }
                          frame #1 {
                            n614 = local write "Current Wavelength (PTI)"(w1049) -> ()
                          }
                        }
                      }
                      frame True {
                        n615 = stacked-sequence {
                          seq-local: [_ w1058 _] -> [_ _ w1064]
                          tunnel: [_ _ w1064] -> w1051
                          tunnel: w1050 -> [_ w1058 _]
                          frame #0 {
                            # "switch to IR\nand recal mono"
                            n616 = One Button Dialog(message="Please switch\nto the IR grating\nnow.") -> (true=w1052:bool)  [unwired: 1 in]
                            n617 = case shown="True" w1052 {
                              frame False {
                              }
                              frame True {
                                n618 = call "UserInputMonoValue.vi"() -> ("Monochromator readout"=w1056:dbl)  [unwired: 17 in, 2 out]
                                n619 = local write "Is IR"(TRUE ("Is IR")) -> ()
                                n620 = Multiply(x=w1056, y=2.0) -> (x*y=w1054:dbl)
                                n621 = local write "Current Wavelength (PTI)"(w1054) -> ()
                              }
                            }
                          }
                          frame #1 {
                            # "now in IR, move \nto new wavelength"
                            n622 = local read "Current Wavelength (PTI)"() -> (w1061:dbl)
                            n623 = Divide(x=w1058, y=2.0) -> (x/y=w1059:dbl)
                            n624 = Divide(x=w1061, y=2.0) -> (x/y=w1060:dbl)
                            n625 = call "ChazMoveMono.vi"("Move to"=w1059, "Current"=w1060) -> ()  [unwired: 8 in, 2 out]
                          }
                          frame #2 {
                            n626 = local write "Current Wavelength (PTI)"(w1064) -> ()
                          }
                        }
                      }
                    }
                  }
                }
              }
              frame #1 {
                n627 = call <vilib>:"General Error Handler.vi"() -> ("error out"=w1065:errorcluster)  [unwired: 11 in, 4 out]
              }
            }
          }
          frame True {
            # "Oriel Mono"
            n628 = call "m_open.vi"() -> ("error out"=w1082:errorcluster, "configuration file path copy"=w1083:path)  [unwired: 2 in]
            n629 = call "GetWave.vi"("error in (no error)"=w1082) -> ("error out"=w1075:errorcluster, "Present Wavelength"=w1071:dbl)  [unwired: 1 in]
            n630 = call "RG Get User Input Wavelength.vi"("Current wavelength"=w1071) -> ("Go to wavelength"=w1070:i32)  [unwired: 10 in]
            n631 = call "getgrat.vi"("error in (no error)"=w1075) -> ("error out"=w1076:errorcluster, "Grating"=→"Grating":i32)  [unwired: 1 in]
            n632 = Less Or Equal?(x=w1070, y=590.0) -> (x <= y?=w1073:bool)
            n633 = Select(t=1.0, s=w1073, f=2.0) -> (s? t:f=w1077:dbl)
            n634 = call "setgrat.vi"("error in (no error)"=w1076, "Grating"=w1077) -> ("error out"=w1074:errorcluster)  [unwired: 1 in]
            n635 = call "gowave.vi"("error in (no error)"=w1074, "Destination Wavelength"=w1070) -> ("error out"=w1069:errorcluster)
            n636 = call "GetWave.vi"("error in (no error)"=w1069) -> ("error out"=w1068:errorcluster, "Present Wavelength"=w1067:dbl)  [unwired: 1 in]
            n637 = local write "Current wavelength (Oriel)"(w1067) -> ()
            n638 = call "m_close.vi"("error in (no error)"=w1068, "configuration file path"=w1083) -> ("error out"=w1072:errorcluster)  [unwired: 1 out]
          }
        }
        n639 = flat-sequence {
          tunnel: w1011 -> [_]
          frame #0 {
            n640 = local write "3 - Move mono"(FALSE ("3 - Move shutter")) -> ()
            n641 = One Button Dialog(message="Wavelength change complete.") -> ()  [unwired: 1 in, 1 out]
          }
        }
      }
    }
  }
